vi "3.2.0_BOOST_MODE.vi"(6 "Data in":T2, 8 "error in (no error)":errorcluster, 9 "AllControls In":T1, 10 "?":T3, 11 "Message Queue out":T4) -> (0 "error out":errorcluster, 1 "Flow":string, 2 "Data":T3, 3 "Message Queue Out":T4, 4 "Data out":T2)   [LabVIEW 2017]
uses:
  Depends/AMC/subVIs/TypeDefs/amc_Message Queue.ctl
  Depends/AMC/subVIs/TypeDefs/amc_Message.ctl
  Depends/Tools/Keyed Array/Tools_KeyedArray KeyedArray.ctl
  Ctrls/Data.ctl
  Ctrls/CSV_Data.ctl
  Ctrls/AllControls.ctl
  DIPC 692 Daemon API/typdef/get_parameter.ctl
  Ctrls/AlarmIndex.ctl
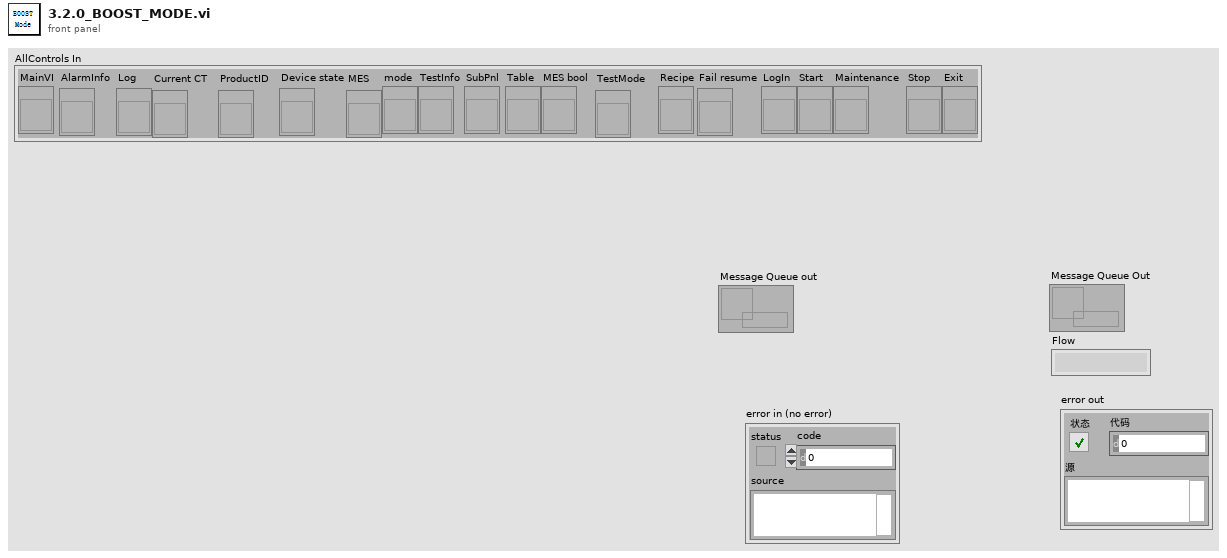
[diagram p1: front panel]
types:
  T1 = typedef "AllControls.ctl" = cluster{"MainVI":refnum<vi>, "AlarmInfo":refnum<vi>, "Log":refnum<vi>, "Current CT":refnum<vi>, "ProductID":refnum<vi>, "Device state":refnum<vi>, "MES":refnum<vi>, "mode":refnum<vi>, "TestInfo":refnum<vi>, "SubPnl":refnum<vi>, "Table":refnum<vi>, "MES bool":refnum<vi>, "TestMode":refnum<vi>, "Recipe":refnum<vi>, "Fail resume":refnum<vi>, "LogIn":refnum<vi>, "Start":refnum<vi>, "Maintenance":refnum<vi>, "Stop":refnum<vi>, "Exit":refnum<vi>}
  T2 = typedef "CSV_Data.ctl" = cluster{"Initialisation":cluster{"LMT - Connect UUT (con COM)":string, "LMT - Software Version (rrel)":string, "LMT - Write SKU file (wskuc)":string, "LMT - SKU file name":string, "Connect UUT DDM":string, "Read DDM EOL Timestamp - Mode":string, "Read DDM EOL Timestamp - Timestamp":string, "Read DDM EOL Timestamp - Rig ID":string, "Read DDM EOL Timestamp - Passmark ID":string, "Read DDM EOL Timestamp - Passmark Rev":string, "Software Version before flashing":string, "Read Hardware Serial":string, "UUT DDM SN":string, "Compare DDM SN with MES SN":string, "Backup PCBA Calibration EEPROM Response - CAL":string, "Flash Firmware Version":string, "Check SW Version":string, "Read DDM SW Version after flashing":string, "Set SKU Config":string, "Ready Status":string, "Set Device Mode to EOL":string, "DDM Parameter - Voltage":string, "DDM Parameter - Current":string, "DDM Parameter - Power":string, "DDM Parameter - Speed":string, "DDM Parameter - Pressure":string, "Tester Parameter - Voltage":string, "Tester Parameter - Current":string, "Tester Parameter - Power":string, "Tester Parameter - Ambient Pressure":string, "Tester Parameter - Ambient Temperature":string, "Calculated Parameter - DDM Pressure Corrected":string, "Calculated Parameter - DDM Real Power":string, "Calculated Parameter - Delta V":string}, "BEMF_Calibration":cluster{"Calibration Result - eol_cold_bemf_temp":string, "DDM Ambient Temp":string, "Restriction Plate Diameter":string, "Calibration Result - eol_bemf_mp_cold_coef_a":string, "Calibration Result - eol_bemf_mp_cold_coef_b":string, "Calibration Result - eol_bemf_mp_cold_coef_c":string, "Calibration Result - eol_bemf_lsi_cold_ref_coeffs":string, "Get - Calibration Result - eol_bemf_lsi_speed":string, "Get - Calibration Result - eol_bemf_lsi_integral_0":string, "Calibration Result - eol_bemf_lsi_integral_1":string, "Get - Calibration Result - eol_bemf_lsi_integral_2":string, "Get - Calibration Result - eol_cold_bemf":string, "Get - Calibration Result - eol_cold_bemf_fisf":string, "Finalise Calibration":string, "Compare -Calibration Result - eol_cold_bemf":string, "Compare -Calibration Result - eol_cold_bemf_fisf":string}, "ECO":cluster{"Reset Power Tune":string, "Reset BEMF FISF Calibration":string, "Restriction Plate Diameter":string, "ECO - Stabilisation Time":string, "ECO - DDM Parameter - Voltage":string, "ECO - DDM Parameter - Current":string, "ECO - DDM Parameter - Power":string, "ECO - DDM Parameter - Measured Power":string, "ECO - DDM Parameter - Speed":string, "ECO - DDM Parameter - Pressure":string, "ECO - Tester Parameter - Voltage":string, "ECO - Tester Parameter - Current":string, "ECO - Tester Parameter - Power":string, "ECO - Tester Parameter - Ambient Pressure":string, "ECO - Tester Parameter - Ambient Temperature":string, "ECO - Tester Parameter - Ambient Humidity":string, "ECO - Calculated Parameter - DDM Pressure Corrected":string, "ECO - Calculated Parameter - DDM Real Power":string, "ECO - Calculated Parameter - Delta V":string, "ECO - Calculated Parameter - Flowrate":string, "ECO - Calculated Parameter - Airwatt":string, "ECO - Formula":string, "PT ECO - Power Tune Mode Status":string}, "BOOST":cluster{"Restriction Plate Diameter":string, "BOOST - Stabilisation Time":string, "BOOST - DDM Parameter - Voltage":string, "BOOST - DDM Parameter - Current":string, "BOOST - DDM Parameter - Power":string, "BOOST - DDM Parameter - Measured Power":string, "BOOST - DDM Parameter - Speed":string, "BOOST - DDM Parameter - Pressure":string, "BOOST - Tester Parameter - Voltage":string, "BOOST - Tester Parameter - Current":string, "BOOST - Tester Parameter - Power":string, "BOOST - Tester Parameter - Ambient Pressure":string, "BOOST - Tester Parameter - Ambient Temperature":string, "BOOST - Tester Parameter - Ambient Humidity":string, "BOOST - Calculated Parameter - DDM Pressure Corrected":string, "BOOST - Calculated Parameter - DDM Real Power":string, "BOOST - Calculated Parameter - Delta V":string, "BOOST - Calculated Parameter - Flowrate":string, "BOOST - Calculated Parameter - Airwatt":string, "BOOST - Get AM Presence":string, "Air Muscle Turn Off Status":string, "BOOST - Air Muscle Calculated Parameter - Airwatt B":string, "BOOST - Air Muscle Calculate Airwatt Delta":string, "PT BOOST - Power Tune Mode Status":string, "Finalise Calibration":string, "ECO - Get AW Calibration value":string, "BOOST - Get AW Calibration value":string}, "MAX":cluster{"Restriction Plate Diameter":string, "MAX - Stabilisation Time":string, "Get Average Delta Tmag (LSIdelta_FISFdelta_LSItmag_FISFtmag_IIRtmag)":string, "Get Average Delta Tmag FISF":string, "MAX - DDM Parameter - Voltage":string, "MAX - DDM Parameter - Current":string, "MAX - DDM Parameter - Power":string, "MAX - DDM Parameter - Measured Power":string, "MAX - DDM Parameter - Speed":string, "MAX - DDM Parameter - Pressure":string, "MAX - Tester Parameter - Voltage":string, "MAX - Tester Parameter - Current":string, "MAX - Tester Parameter - Power":string, "MAX - Tester Parameter - Ambient Pressure":string, "MAX - Tester Parameter - Ambient Temperature":string, "MAX - Tester Parameter - Ambient Humidity":string, "MAX - Calculated Parameter - DDM Pressure Corrected":string, "MAX - Calculated Parameter - DDM Real Power":string, "MAX - Calculated Parameter - Delta V":string, "MAX - Calculated Parameter - Flowrate":string, "MAX - Calculated Parameter - Airwatt":string, "MAX_FISF_Check_Average_Delta_Tmag":string, "MAX - FISF - BEMF Finetune Result":string, "MAX tune - Delta P1":string, "MAX tune - Calculated Parameter - Airwatt":string, "Calculate Delta Airwatts - MAX finetune - Delta P2":string, "MAX finetune - DDM Parameter - Voltage":string, "MAX finetune - DDM Parameter - Current":string, "MAX finetune - DDM Parameter - Power":string, "MAX finetune - DDM Parameter - Measured Power":string, "MAX finetune - DDM Parameter - Speed":string, "MAX finetune - DDM Parameter - Pressure":string, "MAX finetune - Tester Parameter - Voltage":string, "MAX finetune - Tester Parameter - Current":string, "MAX finetune - Tester Parameter - Power":string, "MAX finetune - Tester Parameter - Ambient Pressure":string, "MAX finetune - Tester Parameter - Ambient Temperature":string, "MAX finetune - Tester Parameter - Ambient Humidity":string, "MAX finetune - Calculated Parameter - DDM Pressure Corrected":string, "MAX finetune - Calculated Parameter - DDM Real Power":string, "MAX finetune - Calculated Parameter - Delta V":string, "MAX finetune - Calculated Parameter - Flowrate":string, "MAX finetune - Calculated Parameter - Airwatt":string, "Check Derate Result":string, "Delta Tmag FISF":string, "Get Hot BEMF Result":string, "Calculate delta Pressure":string, "Finalise Calibration":string, "Calculate & Check Delta BEMF":string, "Delta P Airwatts Value":string}, "LL":cluster{"DDM Ambient Temp":string, "Restriction Plate Diameter":string, "LL - DDM Parameter - Voltage":string, "LL - DDM Parameter - Current":string, "LL - DDM Parameter - Power":string, "LL - DDM Parameter - Measured Power":string, "LL - DDM Parameter - Speed":string, "LL - DDM Parameter - Pressure":string, "LL - Tester Parameter - Voltage":string, "LL - Tester Parameter - Current":string, "LL - Tester Parameter - Power":string, "LL - DDM Real Power":string, "LL - Calibrate Task Detect LL":string}, "HL":cluster{"HL - DDM Parameter - Voltage":string, "HL - DDM Parameter - Current":string, "HL - DDM Parameter - Power":string, "HL - DDM Parameter - Measured Power":string, "HL - DDM Parameter - Speed":string, "HL - DDM Parameter - Pressure":string, "HL - Tester Parameter - Voltage":string, "HL - Tester Parameter - Current":string, "HL - Tester Parameter - Power":string, "HL - DDM Real Power":string, "HL - Calibrate Task Detect HL":string}, "LH":cluster{"Restriction Plate Diameter":string, "LH - DDM Parameter - Voltage":string, "LH - DDM Parameter - Current":string, "LH - DDM Parameter - Power":string, "LH - DDM Parameter - Measured Power":string, "LH - DDM Parameter - Speed":string, "LH - DDM Parameter - Pressure":string, "LH - Tester Parameter - Voltage":string, "LH - Tester Parameter - Current":string, "LH - Tester Parameter - Power":string, "LH - DDM Real Power":string, "LH - Calibrate Task Detect LH":string}, "HH":cluster{"HH - DDM Parameter - Voltage":string, "HH - DDM Parameter - Current":string, "HH - DDM Parameter - Power":string, "HH - DDM Parameter - Measured Power":string, "HH - DDM Parameter - Speed":string, "HH - DDM Parameter - Pressure":string, "HH - Tester Parameter - Voltage":string, "HH - Tester Parameter - Current":string, "HH - Tester Parameter - Power":string, "HH - DDM Real Power":string, "HH - Calibrate Task Detect HH":string}, "Inlet Blockage Calibration":cluster{"Inlet Blockage Calibration - DDM Parameter - Voltage":string, "Inlet Blockage Calibration - DDM Parameter - Current":string, "Inlet Blockage Calibration - DDM Parameter - Power":string, "Inlet Blockage Calibration - DDM Parameter - Measured Power":string, "Inlet Blockage Calibration - DDM Parameter - Speed":string, "Inlet Blockage Calibration - DDM Parameter - Pressure":string, "Inlet Blockage Calibration - Tester Parameter - Voltage":string, "Inlet Blockage Calibration - Tester Parameter - Current":string, "Inlet Blockage Calibration - Tester Parameter - Power":string, "Inlet Blockage Calibration - DDM Real Power":string, "Calibration Inlet Blockage_E":string, "Finalise Calibration":string, "Get Task Detect LL":string, "Get Task Detect HL":string, "Get Task Detect LH":string, "Get Task Detect HH":string, "Calibration Inlet Blockage":string, "Calibration eol cold bemf temp":string}, "GOOD":cluster{"GOOD UNIT - Clear EEPROM Error Log":string, "GOOD UNIT - Write Product Timestamp - Mode":string, "GOOD UNIT - Write Product Timestamp - Timestamp":string, "GOOD UNIT - Write Product Timestamp - Rig ID":string, "GOOD UNIT - Write Product Timestamp - Passmark ID":string, "GOOD UNIT - Write Product Timestamp - Passmark Rev":string, "GOOD UNIT - Set Device Mode to PROD":string, "GOOD UNIT - Backup PCBA Calibration EEPROM Response":string, "GOOD UNIT - Check Security Bit":string, "GOOD UNIT - Set Calibration Lock":string, "GOOD UNIT - Get_Calibration_Lock":string, "GOOD UNIT - Disconnect UUT":string}, "NG":cluster{"NG UNIT - Read NVM Error":string, "NG UNIT - Set Device Mode to FCT":string, "NG UNIT - Backup PCBA Calibration EEPROM Response - CAL":string, "NG UNIT - Backup PCBA Calibration EEPROM Response - ERROR":string, "NG UNIT - Backup PCBA Calibration EEPROM Response - USAGE":string, "NG UNIT - Disconnect UUT":string}, "SN":string, "Table":string[][], "Count":cluster{"Total":i32, "OK":i32, "NG":i32, "Yield":dbl}, "Start Time":timestamp, "daemon reference":refnum<k5>, "CT":dbl, "Config":string[][], "OK/NG":bool, "Station ID":string, "MES DDM SN":string, "MES PCBA SN":string, "Retest":string, "Variant":string, "Initialisation_Status":cluster{"LMT - Connect UUT (con COM)":string, "LMT - Software Version (rrel)":string, "LMT - Write SKU file (wskuc)":string, "LMT - SKU file name":string, "Connect UUT DDM":string, "Read DDM EOL Timestamp - Mode":string, "Read DDM EOL Timestamp - Timestamp":string, "Read DDM EOL Timestamp - Rig ID":string, "Read DDM EOL Timestamp - Passmark ID":string, "Read DDM EOL Timestamp - Passmark Rev":string, "Software Version before flashing":string, "Read Hardware Serial":string, "UUT DDM SN":string, "Compare DDM SN with MES SN":string, "Backup PCBA Calibration EEPROM Response - CAL":string, "Flash Firmware Version":string, "Check SW Version":string, "Read DDM SW Version after flashing":string, "Set SKU Config":string, "Ready Status":string, "Set Device Mode to EOL":string, "DDM Parameter - Voltage":string, "DDM Parameter - Current":string, "DDM Parameter - Power":string, "DDM Parameter - Speed":string, "DDM Parameter - Pressure":string, "Tester Parameter - Voltage":string, "Tester Parameter - Current":string, "Tester Parameter - Power":string, "Tester Parameter - Ambient Pressure":string, "Tester Parameter - Ambient Temperature":string, "Calculated Parameter - DDM Pressure Corrected":string, "Calculated Parameter - DDM Real Power":string, "Calculated Parameter - Delta V":string}, "BEMF_Calibration_Status":cluster{"Calibration Result - eol_cold_bemf_temp":string, "DDM Ambient Temp":string, "Restriction Plate Diameter":string, "Calibration Result - eol_bemf_mp_cold_coef_a":string, "Calibration Result - eol_bemf_mp_cold_coef_b":string, "Calibration Result - eol_bemf_mp_cold_coef_c":string, "Calibration Result - eol_bemf_lsi_cold_ref_coeffs":string, "Get - Calibration Result - eol_bemf_lsi_speed":string, "Get - Calibration Result - eol_bemf_lsi_integral_0":string, "Calibration Result - eol_bemf_lsi_integral_1":string, "Get - Calibration Result - eol_bemf_lsi_integral_2":string, "Get - Calibration Result - eol_cold_bemf":string, "Get - Calibration Result - eol_cold_bemf_fisf":string, "Finalise Calibration":string, "Compare -Calibration Result - eol_cold_bemf":string, "Compare -Calibration Result - eol_cold_bemf_fisf":string}, "ECO_Status":cluster{"Reset Power Tune":string, "Reset BEMF FISF Calibration":string, "Restriction Plate Diameter":string, "ECO - Stabilisation Time":string, "ECO - DDM Parameter - Voltage":string, "ECO - DDM Parameter - Current":string, "ECO - DDM Parameter - Power":string, "ECO - DDM Parameter - Measured Power":string, "ECO - DDM Parameter - Speed":string, "ECO - DDM Parameter - Pressure":string, "ECO - Tester Parameter - Voltage":string, "ECO - Tester Parameter - Current":string, "ECO - Tester Parameter - Power":string, "ECO - Tester Parameter - Ambient Pressure":string, "ECO - Tester Parameter - Ambient Temperature":string, "ECO - Tester Parameter - Ambient Humidity":string, "ECO - Calculated Parameter - DDM Pressure Corrected":string, "ECO - Calculated Parameter - DDM Real Power":string, "ECO - Calculated Parameter - Delta V":string, "ECO - Calculated Parameter - Flowrate":string, "ECO - Calculated Parameter - Airwatt":string, "ECO - Formula":string, "PT ECO - Power Tune Mode Status":string}, "BOOST_Status":cluster{"Restriction Plate Diameter":string, "BOOST - Stabilisation Time":string, "BOOST - DDM Parameter - Voltage":string, "BOOST - DDM Parameter - Current":string, "BOOST - DDM Parameter - Power":string, "BOOST - DDM Parameter - Measured Power":string, "BOOST - DDM Parameter - Speed":string, "BOOST - DDM Parameter - Pressure":string, "BOOST - Tester Parameter - Voltage":string, "BOOST - Tester Parameter - Current":string, "BOOST - Tester Parameter - Power":string, "BOOST - Tester Parameter - Ambient Pressure":string, "BOOST - Tester Parameter - Ambient Temperature":string, "BOOST - Tester Parameter - Ambient Humidity":string, "BOOST - Calculated Parameter - DDM Pressure Corrected":string, "BOOST - Calculated Parameter - DDM Real Power":string, "BOOST - Calculated Parameter - Delta V":string, "BOOST - Calculated Parameter - Flowrate":string, "BOOST - Calculated Parameter - Airwatt":string, "BOOST - Get AM Presence":string, "Air Muscle Turn Off Status":string, "BOOST - Air Muscle Calculated Parameter - Airwatt B":string, "BOOST - Air Muscle Calculate Airwatt Delta":string, "PT BOOST - Power Tune Mode Status":string, "Finalise Calibration":string, "ECO - Get AW Calibration value":string, "BOOST - Get AW Calibration value":string}, "MAX_Status":cluster{"Restriction Plate Diameter":string, "MAX - Stabilisation Time":string, "Get Average Delta Tmag (LSIdelta_FISFdelta_LSItmag_FISFtmag_IIRtmag)":string, "Get Average Delta Tmag FISF":string, "MAX - DDM Parameter - Voltage":string, "MAX - DDM Parameter - Current":string, "MAX - DDM Parameter - Power":string, "MAX - DDM Parameter - Measured Power":string, "MAX - DDM Parameter - Speed":string, "MAX - DDM Parameter - Pressure":string, "MAX - Tester Parameter - Voltage":string, "MAX - Tester Parameter - Current":string, "MAX - Tester Parameter - Power":string, "MAX - Tester Parameter - Ambient Pressure":string, "MAX - Tester Parameter - Ambient Temperature":string, "MAX - Tester Parameter - Ambient Humidity":string, "MAX - Calculated Parameter - DDM Pressure Corrected":string, "MAX - Calculated Parameter - DDM Real Power":string, "MAX - Calculated Parameter - Delta V":string, "MAX - Calculated Parameter - Flowrate":string, "MAX - Calculated Parameter - Airwatt":string, "MAX_FISF_Check_Average_Delta_Tmag":string, "MAX - FISF - BEMF Finetune Result":string, "MAX tune - Delta P1":string, "MAX tune - Calculated Parameter - Airwatt":string, "Calculate Delta Airwatts - MAX finetune - Delta P2":string, "MAX finetune - DDM Parameter - Voltage":string, "MAX finetune - DDM Parameter - Current":string, "MAX finetune - DDM Parameter - Power":string, "MAX finetune - DDM Parameter - Measured Power":string, "MAX finetune - DDM Parameter - Speed":string, "MAX finetune - DDM Parameter - Pressure":string, "MAX finetune - Tester Parameter - Voltage":string, "MAX finetune - Tester Parameter - Current":string, "MAX finetune - Tester Parameter - Power":string, "MAX finetune - Tester Parameter - Ambient Pressure":string, "MAX finetune - Tester Parameter - Ambient Temperature":string, "MAX finetune - Tester Parameter - Ambient Humidity":string, "MAX finetune - Calculated Parameter - DDM Pressure Corrected":string, "MAX finetune - Calculated Parameter - DDM Real Power":string, "MAX finetune - Calculated Parameter - Delta V":string, "MAX finetune - Calculated Parameter - Flowrate":string, "MAX finetune - Calculated Parameter - Airwatt":string, "Check Derate Result":string, "Delta Tmag FISF":string, "Get Hot BEMF Result":string, "Calculate delta Pressure":string, "Finalise Calibration":string, "Calculate & Check Delta BEMF":string, "Delta P Airwatts Value":string}, "LL_Status":cluster{"DDM Ambient Temp":string, "Restriction Plate Diameter":string, "LL - DDM Parameter - Voltage":string, "LL - DDM Parameter - Current":string, "LL - DDM Parameter - Power":string, "LL - DDM Parameter - Measured Power":string, "LL - DDM Parameter - Speed":string, "LL - DDM Parameter - Pressure":string, "LL - Tester Parameter - Voltage":string, "LL - Tester Parameter - Current":string, "LL - Tester Parameter - Power":string, "LL - DDM Real Power":string, "LL - Calibrate Task Detect LL":string}, "HL_Status":cluster{"HL - DDM Parameter - Voltage":string, "HL - DDM Parameter - Current":string, "HL - DDM Parameter - Power":string, "HL - DDM Parameter - Measured Power":string, "HL - DDM Parameter - Speed":string, "HL - DDM Parameter - Pressure":string, "HL - Tester Parameter - Voltage":string, "HL - Tester Parameter - Current":string, "HL - Tester Parameter - Power":string, "HL - DDM Real Power":string, "HL - Calibrate Task Detect HL":string}, "LH_Status":cluster{"Restriction Plate Diameter":string, "LH - DDM Parameter - Voltage":string, "LH - DDM Parameter - Current":string, "LH - DDM Parameter - Power":string, "LH - DDM Parameter - Measured Power":string, "LH - DDM Parameter - Speed":string, "LH - DDM Parameter - Pressure":string, "LH - Tester Parameter - Voltage":string, "LH - Tester Parameter - Current":string, "LH - Tester Parameter - Power":string, "LH - DDM Real Power":string, "LH - Calibrate Task Detect LH":string}, "HH_Status":cluster{"HH - DDM Parameter - Voltage":string, "HH - DDM Parameter - Current":string, "HH - DDM Parameter - Power":string, "HH - DDM Parameter - Measured Power":string, "HH - DDM Parameter - Speed":string, "HH - DDM Parameter - Pressure":string, "HH - Tester Parameter - Voltage":string, "HH - Tester Parameter - Current":string, "HH - Tester Parameter - Power":string, "HH - DDM Real Power":string, "HH - Calibrate Task Detect HH":string}, "Inlet Blockage Calibration_Status":cluster{"Inlet Blockage Calibration - DDM Parameter - Voltage":string, "Inlet Blockage Calibration - DDM Parameter - Current":string, "Inlet Blockage Calibration - DDM Parameter - Power":string, "Inlet Blockage Calibration - DDM Parameter - Measured Power":string, "Inlet Blockage Calibration - DDM Parameter - Speed":string, "Inlet Blockage Calibration - DDM Parameter - Pressure":string, "Inlet Blockage Calibration - Tester Parameter - Voltage":string, "Inlet Blockage Calibration - Tester Parameter - Current":string, "Inlet Blockage Calibration - Tester Parameter - Power":string, "Inlet Blockage Calibration - DDM Real Power":string, "Calibration Inlet Blockage_E":string, "Finalise Calibration":string, "Get Task Detect LL":string, "Get Task Detect HL":string, "Get Task Detect LH":string, "Get Task Detect HH":string, "Calibration Inlet Blockage":string, "Calibration eol cold bemf temp":string}, "GOOD_Status":cluster{"GOOD UNIT - Clear EEPROM Error Log":string, "GOOD UNIT - Write Product Timestamp - Mode":string, "GOOD UNIT - Write Product Timestamp - Timestamp":string, "GOOD UNIT - Write Product Timestamp - Rig ID":string, "GOOD UNIT - Write Product Timestamp - Passmark ID":string, "GOOD UNIT - Write Product Timestamp - Passmark Rev":string, "GOOD UNIT - Set Device Mode to PROD":string, "GOOD UNIT - Backup PCBA Calibration EEPROM Response":string, "GOOD UNIT - Check Security Bit":string, "GOOD UNIT - Set Calibration Lock":string, "GOOD UNIT - Get_Calibration_Lock":string, "GOOD UNIT - Disconnect UUT":string}, "NG_Status":cluster{"NG UNIT - Read NVM Error":string, "NG UNIT - Set Device Mode to FCT":string, "NG UNIT - Backup PCBA Calibration EEPROM Response - CAL":string, "NG UNIT - Backup PCBA Calibration EEPROM Response - ERROR":string, "NG UNIT - Backup PCBA Calibration EEPROM Response - USAGE":string, "NG UNIT - Disconnect UUT":string}, "SKU":string, "Plate_Diameter":string, "Alarm":string}
  T3 = typedef "Data.ctl" = cluster{"Initialisation":cluster{"DDM_Parameter":dbl[], "DDM_Parameter_status":bool[], "Get_Tester_Parameter":dbl[], "Get_Tester_Parameter_status":bool[], "Cal_Tester_Parameter":dbl[], "Cal_Tester_Parameter_status":bool[], "sw_version_before_status":bool, "sw_version_after_status":bool, "Set_SKU_Config_With_LMT_status":bool, "FCT_timestamp_status":bool, "LMT_Connect_to_UUT_status":bool}, "BEMF_Calibration":cluster{"Read_ambient_temperature":dbl, "Calibration_Vaule":dbl[], "Calibration_Vaule _B":dbl[], "Calibration_Vaule_status":bool[], "Calibration_Vaule_B_status":bool[]}, "ECO":cluster{"DDM_Parameter":dbl[], "DDM_Parameter_status":bool[], "Get_Tester_Parameter":dbl[], "Get_Tester_Parameter_status":bool[], "Cal_Tester_Parameter":dbl[], "Cal_Tester_Parameter_status":bool[], "DDM_Parameter_after_power_tune":dbl[], "Get_Tester_Parameter_after_power_tune":dbl[], "Cal_Tester_Parameter_after_power_tune":dbl[], "Cal_Tester_Parameter_after_power_tune_status":bool[], "Delta_P":dbl}, "BOOST":cluster{"DDM_Parameter":dbl[], "DDM_Parameter_status":bool[], "Get_Tester_Parameter":dbl[], "Get_Tester_Parameter_status":bool[], "Cal_Tester_Parameter":dbl[], "Cal_Tester_Parameter_status":bool[], "DDM_Parameter_after_power_tune":dbl[], "Get_Tester_Parameter_after_power_tune":dbl[], "Cal_Tester_Parameter_after_power_tune":dbl[], "Cal_Tester_Parameter_after_power_tune_status":bool[], "airwatts_am_off":dbl, "AW_Delta_(AM_on_and_off)":dbl, "AW_Delta_(AM_on_and_off)_Status":bool, "Delta_P":dbl}, "MAX":cluster{"Average_Tmag_Data":cluster{"LSI Delta in degC":dbl, "FISF Delta in degc":dbl, "LSI Tmag in degC":dbl, "Fisf Tmag in degC":dbl, "IIR Tmag in degC":dbl}, "DDM_Parameter":dbl[], "DDM_Parameter_status":bool[], "Get_Tester_Parameter":dbl[], "Get_Tester_Parameter_status":bool[], "Cal_Tester_Parameter":dbl[], "BEMF_Finetune":cluster{"eol_bemf_mp_cold_coef_c":dbl, "eol_cold_bemf_fisf_offset":dbl}, "AW_Tune":cluster{"delta_P1":dbl, "delta_P_Setting":dbl}, "DDM_Parameter_after_Airwatts_Tune":dbl[], "Get_Tester_Parameter_after_Airwatts_Tune":dbl[], "Cal_Tester_Parameter_after_Airwatts_Tune":dbl[], "DDM_Parameter_after_Airwatts_Finetune":dbl[], "Get_Tester_Parameter_after_Airwatts_Finetune":dbl[], "Cal_Tester_Parameter_after_Airwatts_Finetune":dbl[], "AW_Finetune":cluster{"delta_P2":dbl, "delta_P_Setting":dbl}, "Delta_Tmag_after_tune":cluster{"LSI Delta in degC":dbl, "FISF Delta in degc":dbl, "LSI Tmag in degC":dbl, "Fisf Tmag in degC":dbl, "IIR Tmag in degC":dbl}, "Hot Bemf in mV":dbl, "DDM_Pressure":dbl, "Delta_Pressure":dbl, " Cold Bemf in mV":dbl, " delta Bemf":dbl, " delta p":dbl, "Delta_Pressure_status":bool, " delta Bemf_status":bool, "LSI Delta in degC_status":bool, "FISF Delta in degc_status":bool, "Max_check_derate_status_status":bool, "Average_All_data":dbl[][], "Average_Tmag_Data_status":bool[], "Average_Tmag_Data_after_tune_status":bool[], "Cal_Tester_Parameter_status":bool[], "Cal_Tester_Parameter_status_after_Airwatts_Tune":bool[], "Cal_Tester_Parameter_status_after_Airwatts_FineTune":bool[]}, "Task_Detect_Calib":cluster{"LL":cluster{"DDM_Parameter":dbl[], "DDM_Parameter_status":bool[], "Get_Tester_Parameter":dbl[], "Get_Tester_Parameter_status":bool[], "Set_task_detect_A":dbl, "Set_task_detect_A_Status":bool}, "HL":cluster{"DDM_Parameter":dbl[], "DDM_Parameter_status":bool[], "Get_Tester_Parameter":dbl[], "Get_Tester_Parameter_status":bool[], "Set_task_detect_B":dbl, "Set_task_detect_B_Status":bool}, "LH":cluster{"DDM_Parameter":dbl[], "DDM_Parameter_status":bool[], "Get_Tester_Parameter":dbl[], "Get_Tester_Parameter_status":bool[], "Set_task_detect_C":dbl, "Set_task_detect_C_Status":bool}, "HH":cluster{"DDM_Parameter":dbl[], "DDM_Parameter_status":bool[], "Get_Tester_Parameter":dbl[], "Get_Tester_Parameter_status":bool[], "Set_task_detect_D":dbl, "Read_and_check_calibration_Status":bool[], "Set_task_detect_D_Status":bool}, "Get_eol_inlet_blockage_E":dbl, "Calib_vaule":cluster{"Get_task_detect_LL":dbl, "Get_task_detect_HL":dbl, "Get_task_detect_LH":dbl, "Get_task_detect_HH":dbl, "eol_inlet_blockage":dbl, "eol_code_bemf_temp":dbl}, "calibrated temp":dbl, "Inlet_Blockage_Calibration":cluster{"DDM_Parameter":dbl[], "DDM_Parameter_status":bool[], "Get_Tester_Parameter":dbl[], "Get_Tester_Parameter_status":bool[]}, "Get_eol_inlet_blockage_E_Status":bool}, "good":cluster{"Write_Product_TS":cluster{"TIMESTAMP":i64, "RIG_ID":i64, "PASSMARK_ID":i64, "PASSMARK_REV":i64}, "Read_Product_TS":cluster{"TIMESTAMP":i64, "RIG_ID":i64, "PASSMARK_ID":i64, "PASSMARK_REV":i64}, "Good_Check_Secuity_Bit_Stauts":bool}}
  T4 = typedef "amc_Message Queue.ctl" = refnum<queue>
  T5 = typedef "HD Config.ctl" = cluster{" PC":cluster{"PC Address":u8[], "PC Port":i32}, "FCO":cluster{"COM":refnum<visa-resource-name>, "Baudrate":u32}, "DC Power ":cluster{"COM":refnum<visa-resource-name>, "Baudrate":u32}, "PW3336":cluster{"COM":refnum<visa-resource-name>, "Baudrate":u32}, "Lefoo":cluster{"COM":refnum<visa-resource-name>, "Baudrate":u32}, "AI Model":cluster{"COM":refnum<visa-resource-name>, "Baudrate":u32}, "DIPC":cluster{"COM":refnum<visa-resource-name>}, "NFC":cluster{"IP Address":string, "Port":u16, "Retry":u16}, "Motor":cluster{"COM":refnum<visa-resource-name>, "Baudrate":u32}, "Fail_resume_mode":bool, "GRR":bool}
  T6 = typedef "AlarmIndex.ctl" = enum16{"E-Stop", "Safety light grid", "UUT Sealing Cylinder HomePoint", "UUT Sealing Cylinder WorkPoint", "Orifice fixed Cylinder L HomePoint", "Orifice fixed Cylinder L WorkPoint", "Orifice fixed Cylinder R HomePoint", "Orifice fixed Cylinder R WorkPoint", "UUT Cylinder HomePoint", "UUT Cylinder WorkPoint", "Carrier fixed Cylinder L HomePoint", "Carrier fixed Cylinder L WorkPoint", "Carrier fixed Cylinder R HomePoint", "Carrier fixed Cylinder R WorkPoint", "Probe Cylinder HomePoint", "Probe Cylinder WorkPoint", "Motor Error", "Test Error"}
  T7 = typedef "get_parameter.ctl" = string
  T8 = typedef "Position Config.ctl" = cluster{"OrificeSize_12.7":i32, "OrificeSize_13":i32, "OrificeSize_30":i32, "OrificeSize_16":i32}
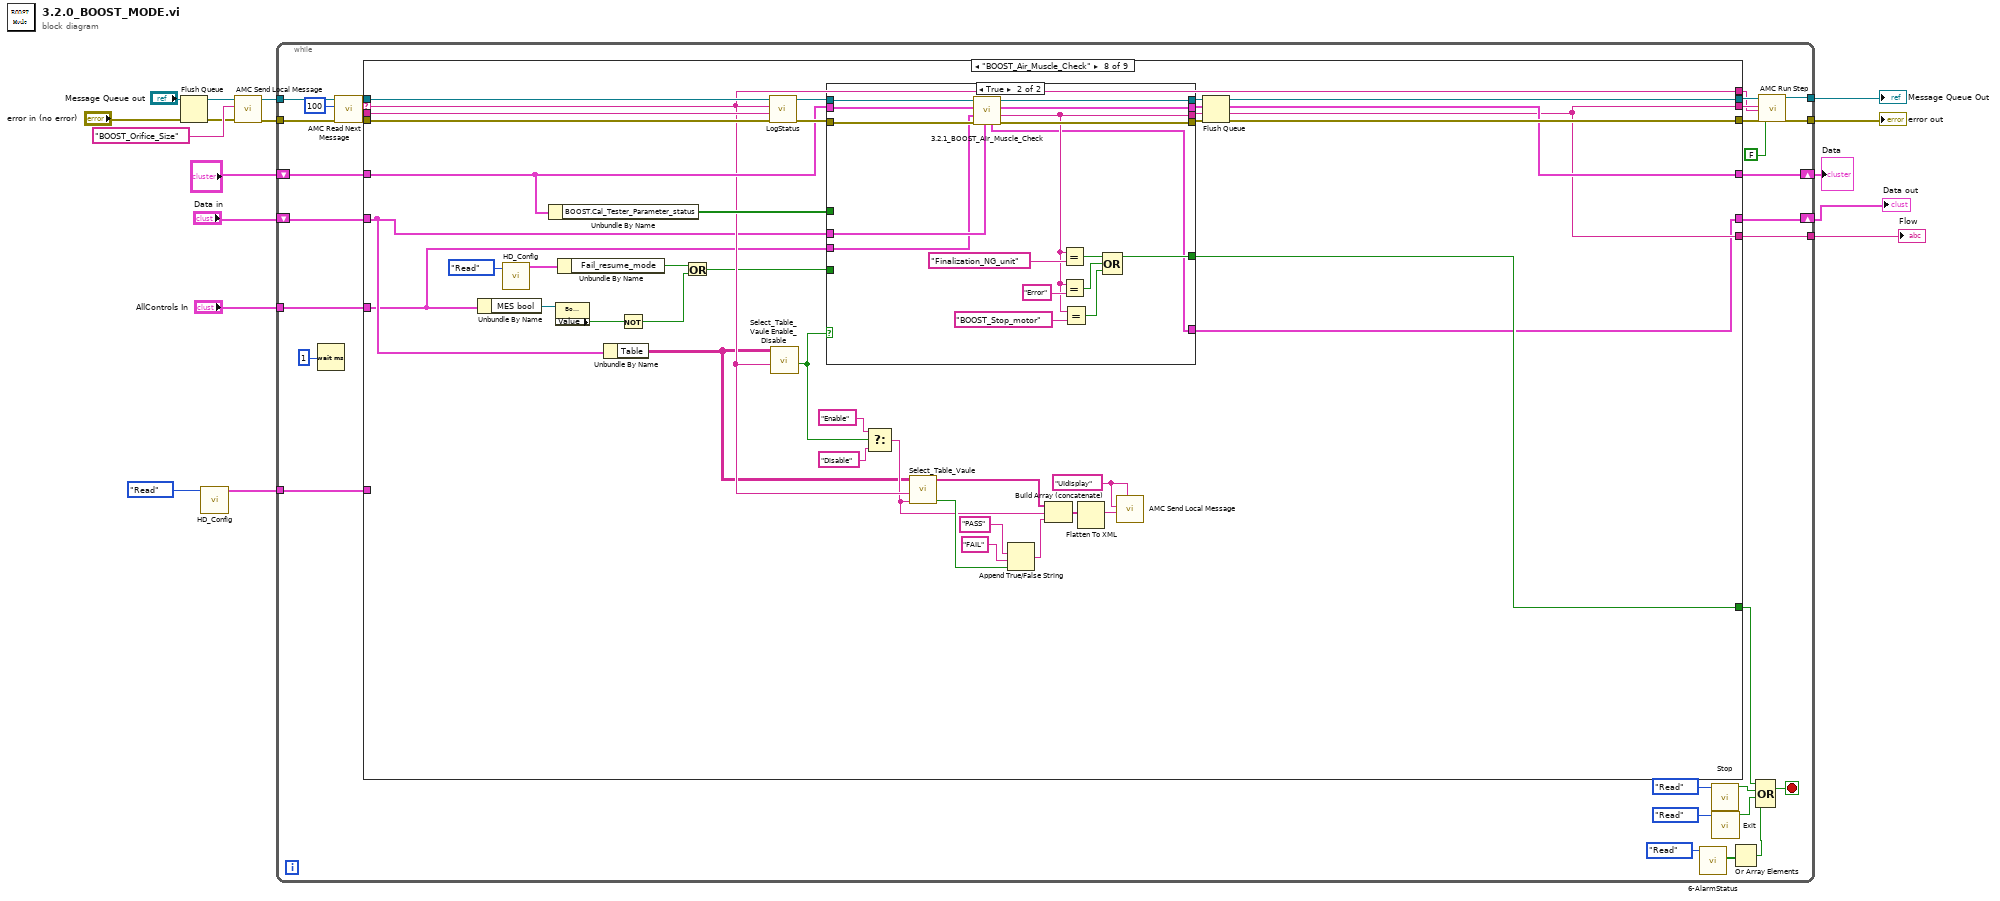
[diagram p0: block diagram]
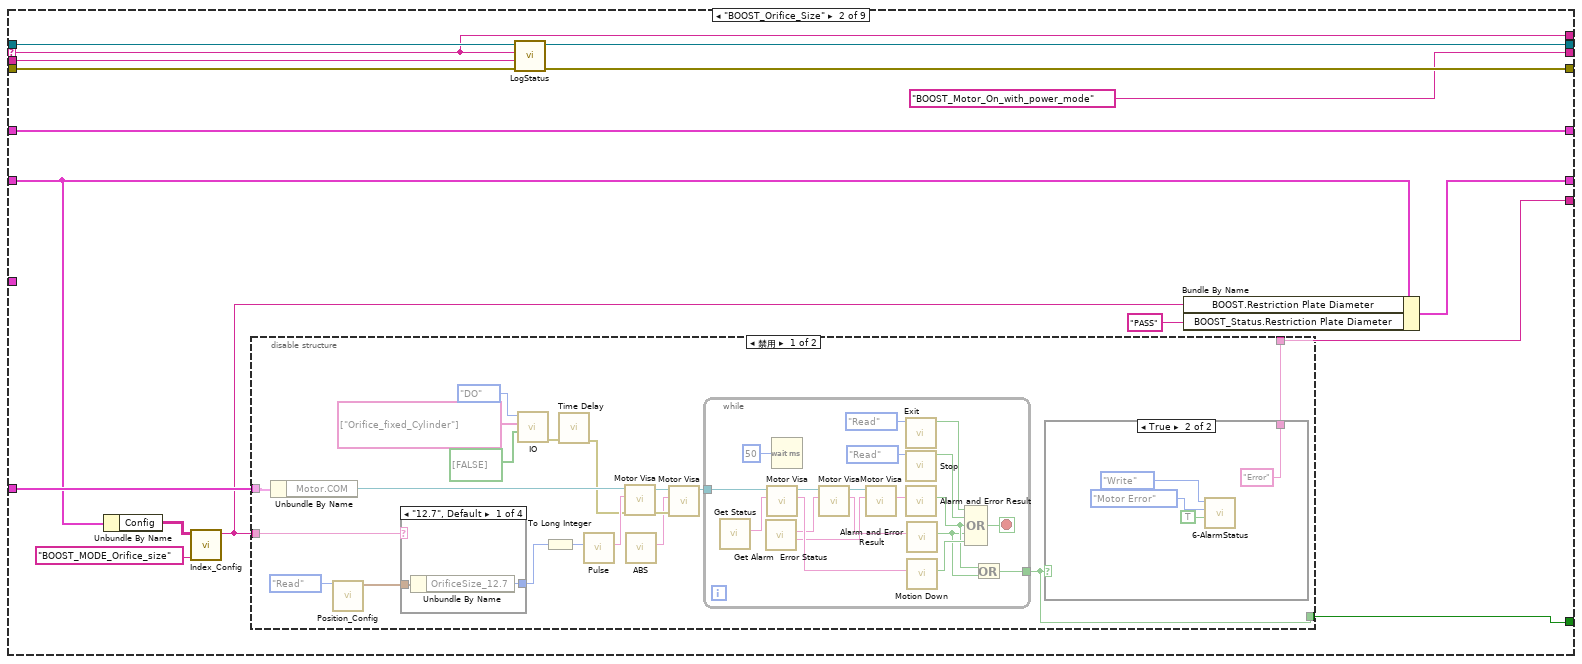
[diagram p3: hidden frame]
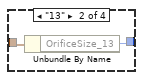
[diagram p4: hidden frame]
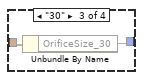
[diagram p5: hidden frame]
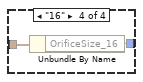
[diagram p6: hidden frame]
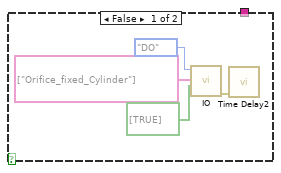
[diagram p7: hidden frame]
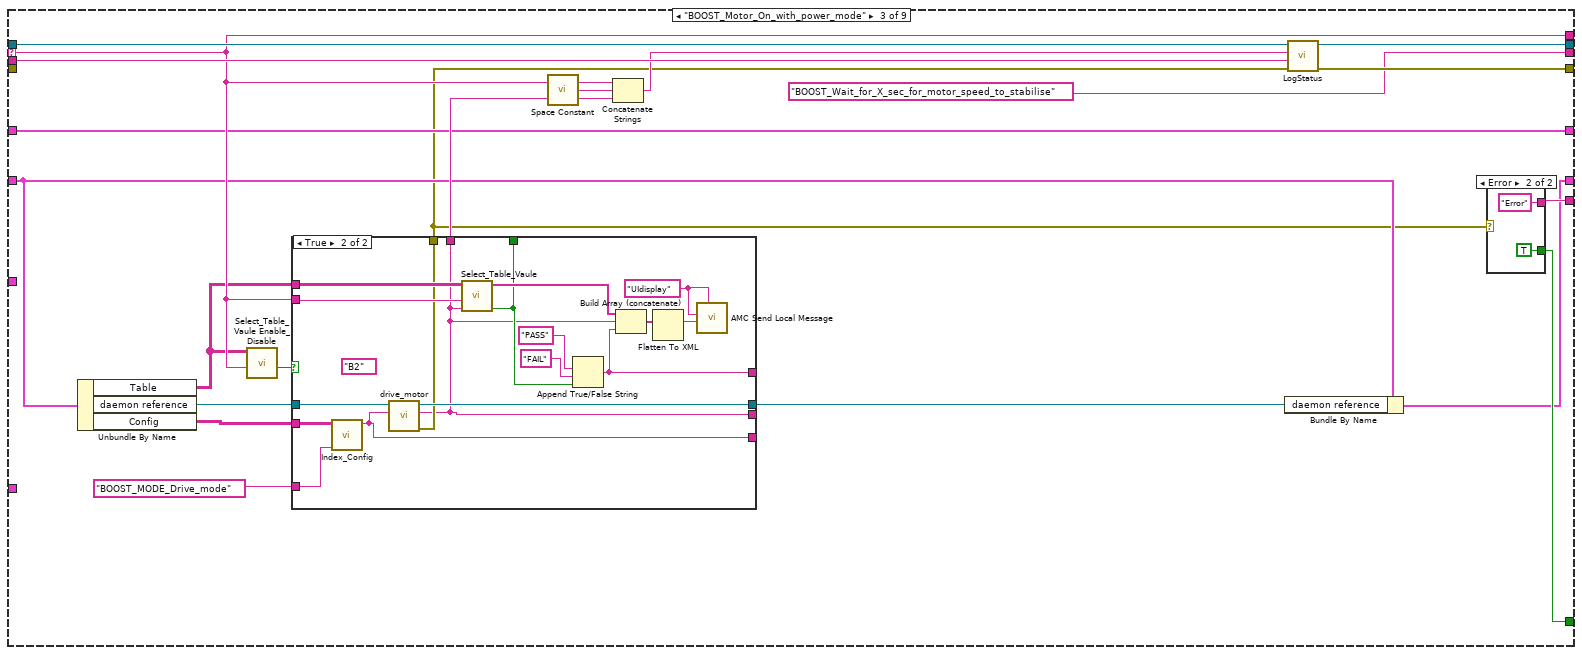
[diagram p9: hidden frame]
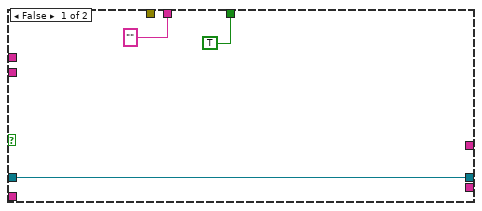
[diagram p11: hidden frame]
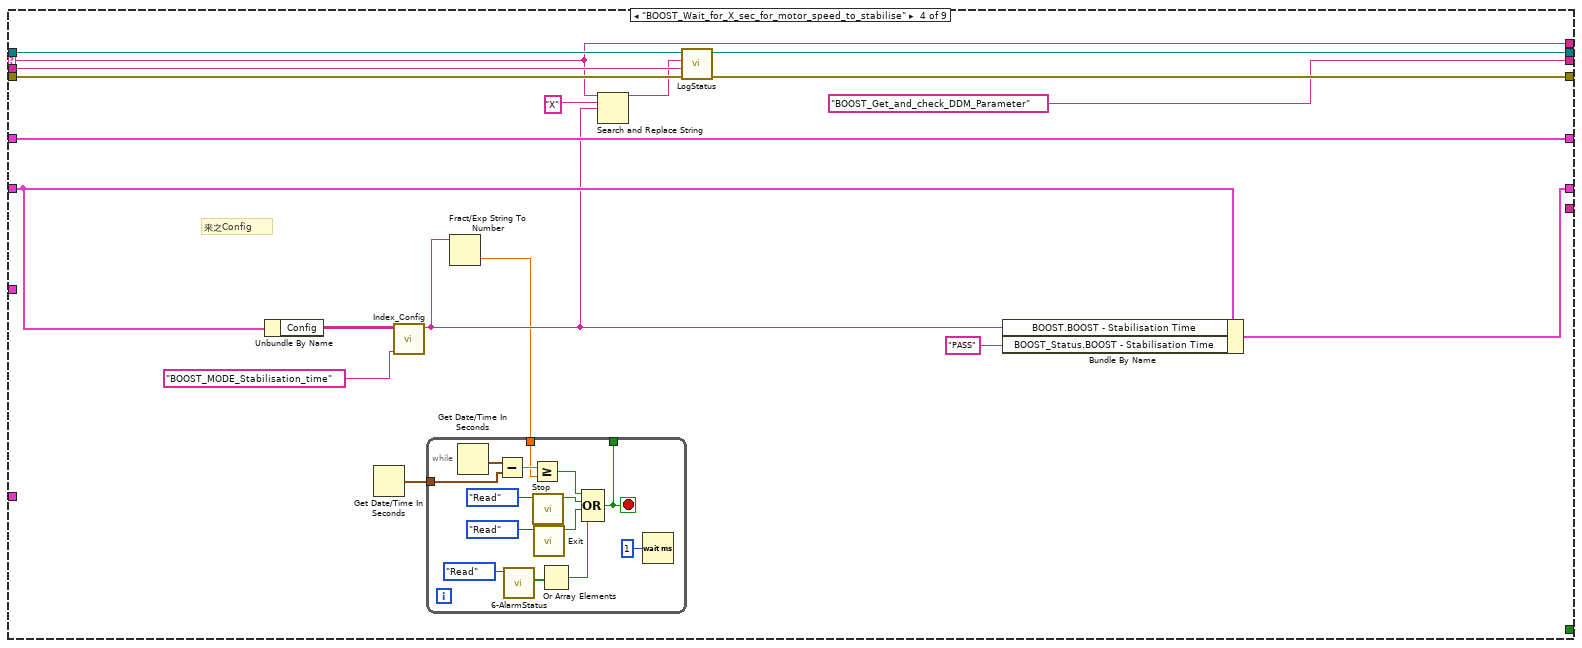
[diagram p12: hidden frame]
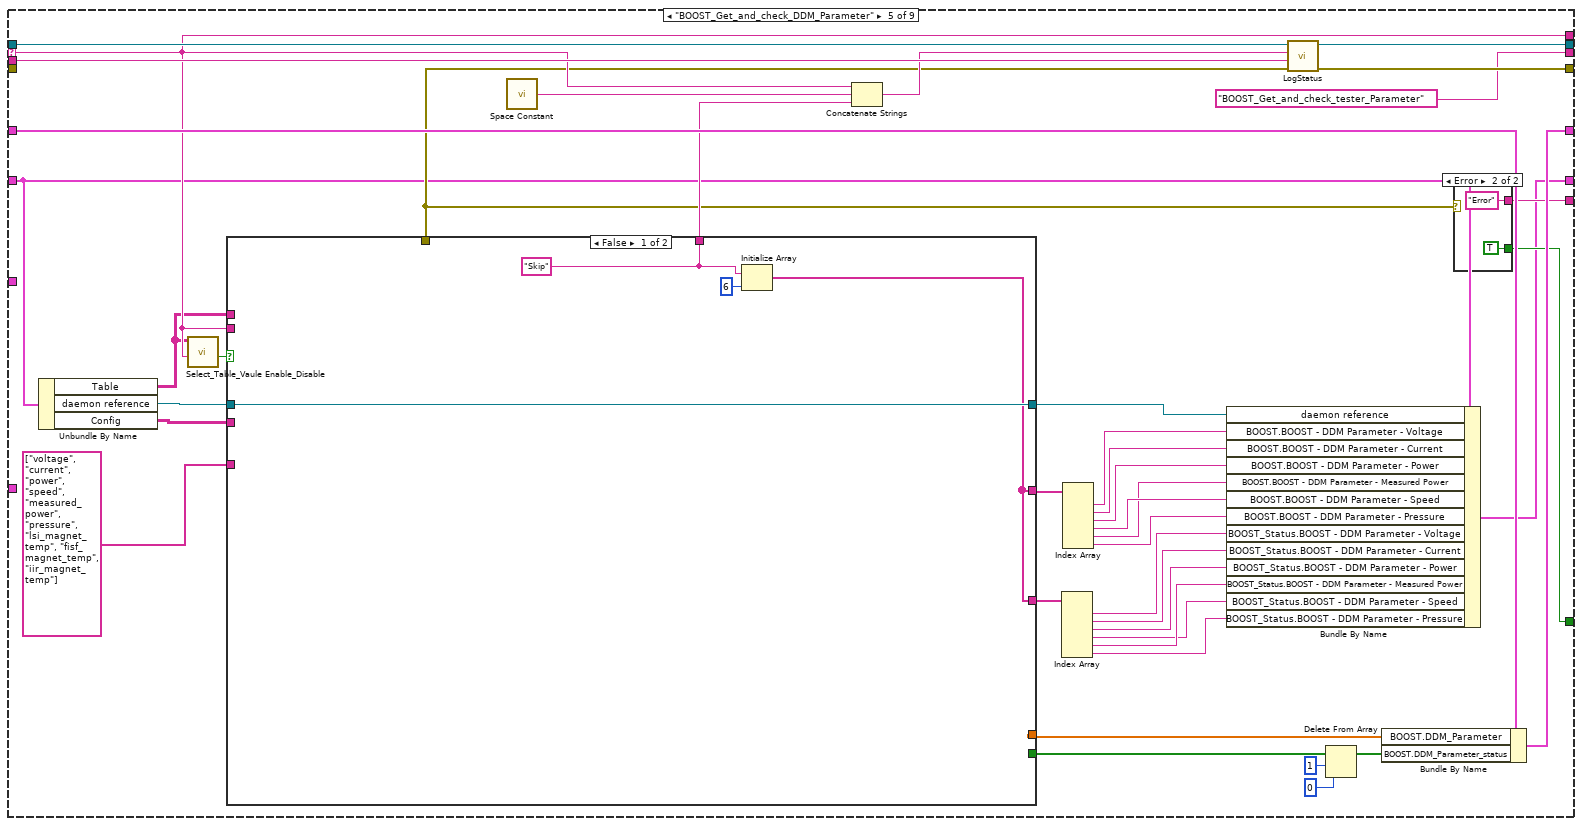
[diagram p13: hidden frame]
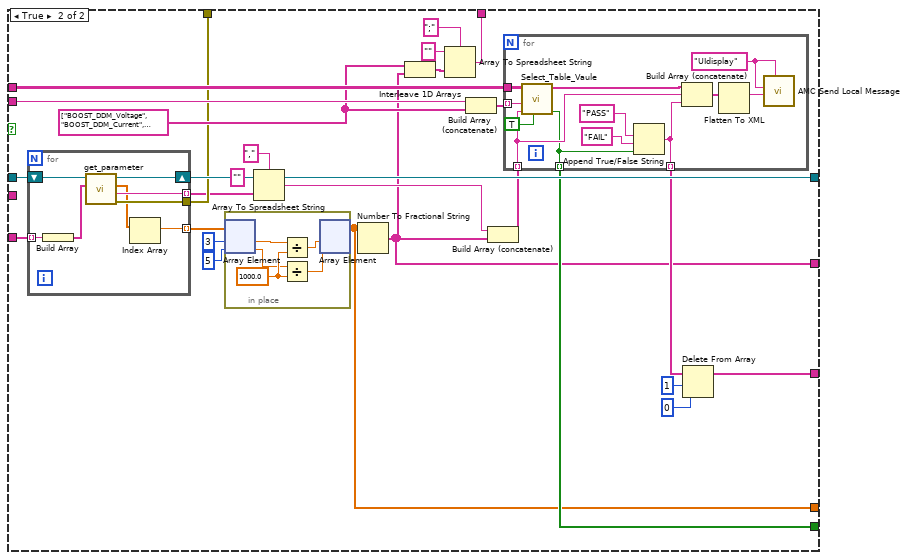
[diagram p15: hidden frame]
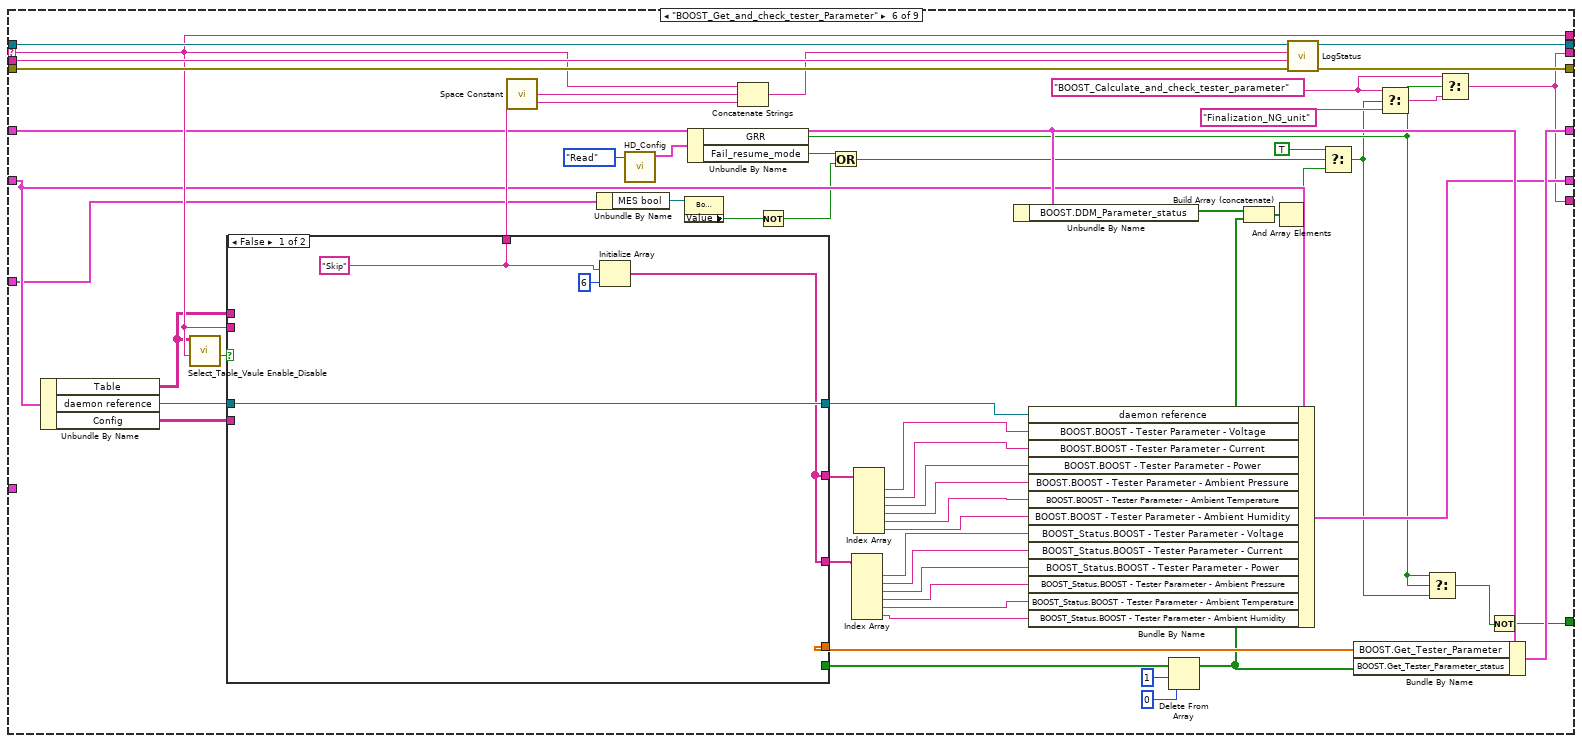
[diagram p16: hidden frame]
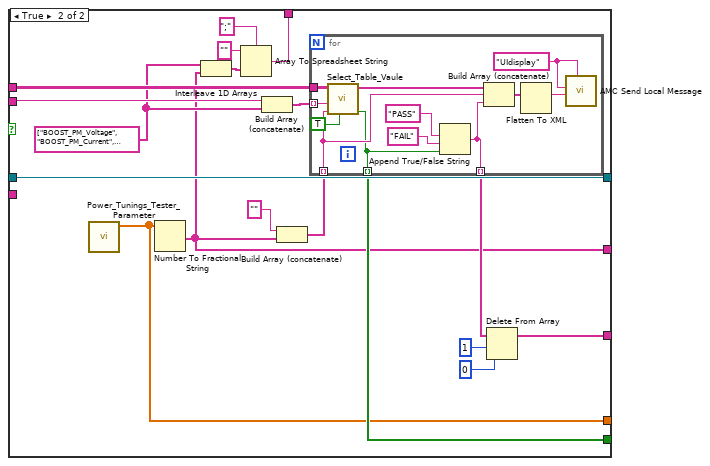
[diagram p17: hidden frame]
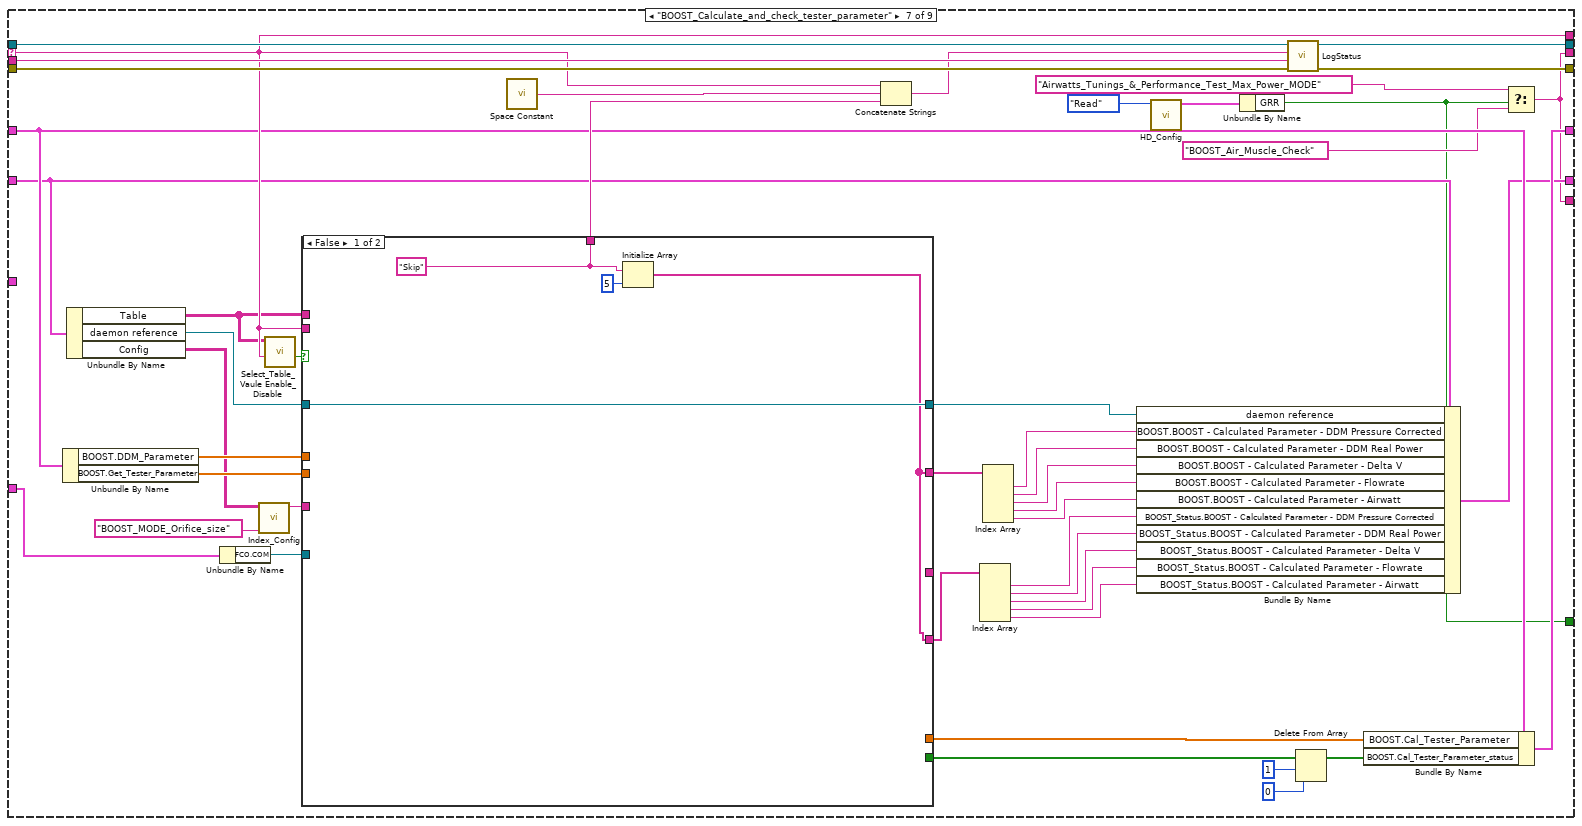
[diagram p18: hidden frame]
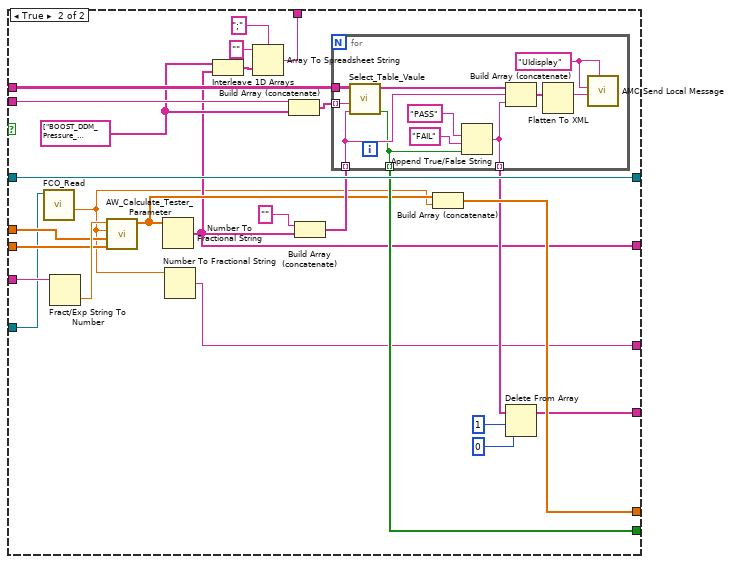
[diagram p19: hidden frame]
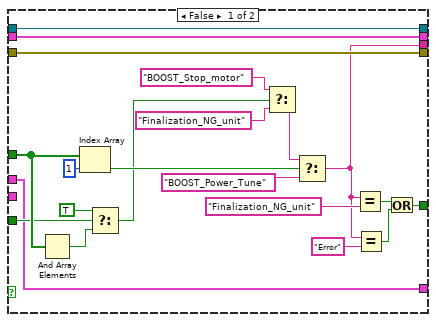
[diagram p20: hidden frame]
diagram:
  n1 = Flush Queue(queue="Message Queue out") -> (queue out=w4:T4)  [unwired: 1 in, 2 out]
  n2 = call "HD_Config.vi"("Step"=enum16{"Initial", "Write", "Read"}."Read") -> ("HD Config out"=w8:T5)  [unwired: 9 in, 1 out]
  n3 = call "AMC Send Local Message.vi"("error in (no error)"="error in (no error)", "Message Name"="BOOST_Orifice_Size", "Message Queue in"=w4) -> ("error out"=w13:errorcluster, "Message Queue out"=w14:T4)  [unwired: 7 in]
  n4 = while {
    tunnel: w14 -> [w47]
    tunnel: [w43] -> w6
    tunnel: w13 -> [w41]
    tunnel: [w38] -> w5
    shift-right: [w34] -> w10
    shift-left: "?" -> [w35]
    tunnel: w8 -> [w33]
    tunnel: [w29] -> w7
    shift-right: [w20] -> w1
    shift-left: "Data in" -> [w22]
    tunnel: "AllControls In" -> [w21]
    stop <- w23 stop-if-true
    n5 = Wait (ms)(milliseconds to wait=u32 1 ("等待时间（毫秒）")) -> ()  [unwired: 1 out]
    n6 = call "AMC Read Next Message.vi"("error in (no error)"=w41, "timeout (1ms)"=100, "Message Queue in"=w47) -> ("error out"=w40:errorcluster, "Message Value"=w31:string, "Message Name"=w45:string, "Message Queue out"=w46:T4)  [unwired: 1 in, 4 out]
    n7 = case shown="\"BOOST_Air_Muscle_Check\"" w45 {
      selector: w45 -> [_ w63 w134 w174 w225 w339 w420 w486 w560]
      tunnel: w46 -> [w51 w67 w141 w180 w234 w348 w428 w501 w574]
      tunnel: [w51 w67 w141 w180 w234 w348 w428 w481 w554] -> w44
      tunnel: w40 -> [w50 w66 _ w179 _ w347 w427 w505 w578]
      tunnel: [w50 w65 w140 w178 w233 w346 w426 w502 w575] -> w39
      tunnel: [_ w60 w128 _ w214 w331 w394 w496 TRUE] -> w24
      tunnel: w35 -> [w49 w56 w126 w170 w230 w334 w417 w497 w570]
      tunnel: [w49 w56 w126 w170 w229 w343 w424 w499 w572] -> w34
      tunnel: w31 -> [_ w64 w139 w177 w232 w345 w425 w504 w577]
      tunnel: [_ w63 w134 w174 w225 w339 w420 w486 w560] -> w30
      tunnel: w33 -> [_ w61 _ _ _ _ w407 _ _]
      tunnel: [_ "BOOST_Motor_On_with_power_mode" "BOOST_Wait_for_X_sec_for_motor_speed_to_stabilise" "BOOST_Get_and_check_DDM_Parameter" "BOOST_Get_and_check_tester_Parameter" w310 w395 w498 w571] -> w32
      tunnel: [_ w59 w129 _ w215 w310 w395 w498 w571] -> w29
      tunnel: w22 -> [w48 w53 w125 w169 w211 w325 w403 w472 w546]
      tunnel: w21 -> [_ _ _ _ _ w313 _ w470 w544]
      tunnel: [w48 w55 w123 w168 w209 w322 w402 w471 w545] -> w20
      frame "假", Default {
      }
      frame "BOOST_Orifice_Size" {
        n8 = Unbundle By Name(w53) -> ("Config"=w58:string[][])
        n9 = call "Index_Config.vi"("Action"="BOOST_MODE_Orifice_size", "config"=w58) -> ("data"=w54:string)  [unwired: 9 in]
        n10 = disable-structure shown="禁用" {
          disable-tunnel: w61 -> [w76 _]
          disable-tunnel: [w75 _] -> w60
          disable-tunnel: [w69 _] -> w59
          disable-tunnel: w54 -> [w68 _]
          frame Disabled {
            n11 = Unbundle By Name(w76) -> ("Motor.COM"=w81:refnum<visa-resource-name>)
            n12 = call "Position_Config.vi"("Step"=enum16{"Initial", "Write", "Read"}."Read") -> ("Position Config out"=w78:T8)  [unwired: 9 in, 1 out]
            n13 = case shown="\"12.7\", Default" w68 {
              tunnel: w78 -> [w88 w90 w92 w94]
              tunnel: [w87 w89 w91 w93] -> w77
              frame "12.7", Default {
                n14 = Unbundle By Name(w88) -> ("OrificeSize_12.7"=w87:i32)
              }
              frame "13" {
                n15 = Unbundle By Name(w90) -> ("OrificeSize_13"=w89:i32)
              }
              frame "30" {
                n16 = Unbundle By Name(w92) -> ("OrificeSize_30"=w91:i32)
              }
              frame "16" {
                n17 = Unbundle By Name(w94) -> ("OrificeSize_16"=w93:i32)
              }
            }
            n18 = call "IO.vi"("DO DATA"=bool[] [FALSE] ("Writel_IO"), "IO Name"=string[] ["Orifice_fixed_Cylinder"], "IO?"=enum16{"DI", "DO"}."DO") -> ("error out"=w71:errorcluster)  [unwired: 7 in, 1 out]
            n19 = To Long Integer(number=w77) -> (32bit integer=w83:i32)
            n20 = call "Time Delay"("error in (no error)"=w71) -> ("error out"=w70:errorcluster)  [unwired: 10 in]
            n21 = call "Pulse.vi"("Pulse"=w83) -> ("Pulse"=w84:string)  [unwired: 10 in]
            n22 = call "Motor Visa.vi"("错误输入（无错误）"=w70, "Command"=w84, "VISA资源名称"=w81) -> ("错误输出"=w85:errorcluster, "VISA资源名称输出"=w86:refnum<visa-resource-name>)  [unwired: 6 in, 1 out]
            n23 = call "ABS.vi"() -> ("绝对模式"=w82:string)  [unwired: 11 in]
            n24 = call "Motor Visa.vi"("错误输入（无错误）"=w85, "Command"=w82, "VISA资源名称"=w86) -> ("VISA资源名称输出"=w80:refnum<visa-resource-name>)  [unwired: 6 in, 2 out]
            n25 = while {
              tunnel: w80 -> [w120]
              tunnel: [w103] -> w75
              stop <- w110 stop-if-true
              n26 = call "Get Status.vi"() -> ("Command"=w121:string)  [unwired: 11 in]
              n27 = call "Get Alarm  Error Status.vi"() -> ("AlarmStatus"=w113:string, "ErrorStatus"=w114:string)  [unwired: 10 in]
              n28 = call "Motor Visa.vi"("Command"=w121, "VISA资源名称"=w120) -> ("读取缓冲区"=w119:string, "VISA资源名称输出"=w112:refnum<visa-resource-name>)  [unwired: 7 in, 1 out]
              n29 = Wait (ms)(milliseconds to wait=u32 50 ("等待时间（毫秒）")) -> ()  [unwired: 1 out]
              n30 = call "Motor Visa.vi"("Command"=w114, "VISA资源名称"=w112) -> ("读取缓冲区"=w116:string, "VISA资源名称输出"=w117:refnum<visa-resource-name>)  [unwired: 7 in, 1 out]
              n31 = call "Motor Visa.vi"("Command"=w113, "VISA资源名称"=w117) -> ("读取缓冲区"=w115:string)  [unwired: 7 in, 2 out]
              n32 = call "Exit.vi"("Step"=enum16{"Initial", "Write", "Read"}."Read" ("step")) -> ("Exit Out"=w106:bool)  [unwired: 9 in, 1 out]
              n33 = call "Stop.vi"("Step"=enum16{"Initial", "Write", "Read"}."Read") -> ("Stop Out"=w107:bool)  [unwired: 9 in, 1 out]
              n34 = call "Alarm and Error Result.vi"("Command"=w115) -> ("Alarm or Error"=w105:bool)  [unwired: 10 in]
              n35 = call "Alarm and Error Result.vi"("Command"=w116) -> ("Alarm or Error"=w104:bool)  [unwired: 10 in]
              n36 = call "Motion Down.vi"("Command"=w119) -> ("Motion Down"=w111:bool)  [unwired: 10 in]
              n37 = Compound Arithmetic op=OR(w106, w107, w105, w104, w111) -> (w110:bool)
              n38 = Or(x=w105, y=w104) -> (x .or. y?=w103:bool)
            }
            n39 = case shown="True" w75 {
              tunnel: [_ "Error" ("Message Name")] -> w69
              frame False {
                n40 = call "IO.vi"("DO DATA"=bool[] [TRUE] ("Writel_IO"), "IO Name"=string[] ["Orifice_fixed_Cylinder"], "IO?"=enum16{"DI", "DO"}."DO") -> ("error out"=w98:errorcluster)  [unwired: 7 in, 1 out]
                n41 = call "Time Delay2"("error in (no error)"=w98) -> ()  [unwired: 10 in, 1 out]
              }
              frame True {
                n42 = call "6-AlarmStatus.vi"("AlarmValue"=TRUE, "AlarmIndex"=AlarmIndex."Motor Error", "Step"=enum16{"Initial", "Write", "Read"}."Write") -> ()  [unwired: 7 in, 2 out]
              }
            }
          }
          frame Enabled {
          }
        }
        n43 = call "LogStatus.vi"("error in (no error)"=w66, "last message"=w64, "message"=w63) -> ("error  out"=w65:errorcluster)  [unwired: 8 in]
        n44 = Bundle By Name(cluster=w53, "BOOST.Restriction Plate Diameter"=w54, "BOOST_Status.Restriction Plate Diameter"="PASS") -> (w55:T2)
      }
      frame "BOOST_Motor_On_with_power_mode" {
        n45 = Unbundle By Name(w125) -> ("Table"=w133:string[][], "daemon reference"=w138:refnum<k5>, "Config"=w131:string[][])
        n46 = call "Select_Table_Vaule Enable_Disable.vi"("Action"=w134, "Table"=w133) -> ("Enable"=w135:bool)  [unwired: 8 in, 1 out]
        n47 = case shown="True" w135 {
          tunnel: w138 -> [w145 w163]
          tunnel: [TRUE w153] -> _
          tunnel: [w145 w157] -> w122
          tunnel: ["" ("response") w149] -> w127
          tunnel: w134 -> [_ w156]
          tunnel: w133 -> [_ w155]
          tunnel: w131 -> [_ w152]
          tunnel: "BOOST_MODE_Drive_mode" -> [_ w151]
          tunnel: [_ w150] -> w124
          tunnel: [_ w149] -> _
          tunnel: [_ w148] -> _
          tunnel: [_ w147] -> _
          frame False {
          }
          frame True {
            (unwired) "B2" ("Power Mode")
            w162 = "UIdisplay" ("Process (\"\" - local)")
            n48 = call "Index_Config.vi"("Action"=w151, "config"=w152) -> ("data"=w147:string)  [unwired: 9 in]
            n49 = call "drive_motor.vi"("Power Mode"=w147, "daemon reference in"=w163) -> ("error out"=w150:errorcluster, "response"=w149:string, "daemon reference out"=w157:refnum<k5>)  [unwired: 6 in, 1 out]
            n50 = call "Select_Table_Vaule.vi"("Vaule"=w149, "Action"=w156, "Table"=w155) -> ("Result"=w153:bool, "vaule"=w154:string[])  [unwired: 7 in]
            n51 = Append True/False String(1:w153, 2:"FAIL" ("真字符串"), 3:"PASS" ("真字符串")) -> (0:w148:string)  [unwired: 1 in]
            n52 = Build Array (concatenate)(w154, w149, w148) -> (w161:string[])
            n53 = Flatten To XML(anything=w161) -> (xml string=w160:string)
            n54 = call "AMC Send Local Message.vi"("Process (\"\" - local)"=w162, "Message Value"=w160, "Message Name"=w162) -> ()  [unwired: 7 in, 2 out]
          }
        }
        n55 = call <vilib>:"Space Constant.vi"() -> ("String"=w137:string)
        n56 = Concatenate Strings(w134, w137, w127) -> (w136:string)
        n57 = Bundle By Name(cluster=w125, "daemon reference"=w122) -> (w123:T2)
        n58 = call "LogStatus.vi"("error in (no error)"=w124, "last message"=w139, "message"=w136) -> ("error  out"=w140:errorcluster)  [unwired: 8 in]
        n59 = case shown="Error" w124 {
          tunnel: [_ TRUE] -> w128
          tunnel: [_ "Error"] -> w129
          frame No Error {
          }
          frame Error {
          }
        }
      }
      frame "BOOST_Wait_for_X_sec_for_motor_speed_to_stabilise" {
        # "来之Config"
        n60 = Unbundle By Name(w169) -> ("Config"=w172:string[][])
        n61 = Get Date/Time In Seconds() -> (seconds since 1Jan1904=w166:timestamp)
        n62 = call "Index_Config.vi"("Action"="BOOST_MODE_Stabilisation_time", "config"=w172) -> ("data"=w167:string)  [unwired: 9 in]
        n63 = Fract/Exp String To Number(string=w167) -> (number=w165:dbl)  [unwired: 3 in, 1 out]
        n64 = while {
          tunnel: w166 -> [w187]
          tunnel: w165 -> [w184]
          tunnel: [w183] -> _
          stop <- w183 stop-if-true
          n65 = Get Date/Time In Seconds() -> (seconds since 1Jan1904=w188:timestamp)
          n66 = Subtract(x=w188, y=w187) -> (x-y=w186:dbl)
          n67 = call "6-AlarmStatus.vi"("Step"=enum16{"Initial", "Write", "Read"}."Read") -> ("AlarmValue Out"=w191:bool[])  [unwired: 9 in, 1 out]
          n68 = Greater Or Equal?(x=w186, y=w184) -> (x >= y?=w185:bool)
          n69 = call "Stop.vi"("Step"=enum16{"Initial", "Write", "Read"}."Read") -> ("Stop Out"=w189:bool)  [unwired: 9 in, 1 out]
          n70 = call "Exit.vi"("Step"=enum16{"Initial", "Write", "Read"}."Read" ("step")) -> ("Exit Out"=w193:bool)  [unwired: 9 in, 1 out]
          n71 = Or Array Elements(Boolean array=w191) -> (logical OR=w190:bool)
          n72 = Compound Arithmetic op=OR(w185, w189, w193, w190) -> (w183:bool)
          n73 = Wait (ms)(milliseconds to wait=u32 1 ("等待时间（毫秒）")) -> ()  [unwired: 1 out]
        }
        n74 = Search and Replace String(input string=w174, search string="X" ("搜索字符串"), replace string=w167) -> (result string=w175:string)  [unwired: 5 in, 3 out]
        n75 = call "LogStatus.vi"("error in (no error)"=w179, "last message"=w177, "message"=w175) -> ("error  out"=w178:errorcluster)  [unwired: 8 in]
        n76 = Bundle By Name(cluster=w169, "BOOST.BOOST - Stabilisation Time"=w167, "BOOST_Status.BOOST - Stabilisation Time"="PASS") -> (w168:T2)
      }
      frame "BOOST_Get_and_check_DDM_Parameter" {
        n77 = Unbundle By Name(w211) -> ("Table"=w224:string[][], "daemon reference"=w231:refnum<k5>, "Config"=w222:string[][])
        n78 = call "Select_Table_Vaule Enable_Disable.vi"("Action"=w225, "Table"=w224) -> ("Enable"=w223:bool)  [unwired: 8 in, 1 out]
        n79 = case shown="False" w223 {
          tunnel: w231 -> [w240 w266]
          tunnel: [w240 w265] -> w210
          tunnel: [w239 w257] -> w226
          tunnel: w225 -> [_ w262]
          tunnel: w224 -> [_ w267]
          tunnel: w222 -> [_ _]
          tunnel: [_ w251] -> w220
          tunnel: [_ w264] -> w219
          tunnel: [_ w255] -> w212
          tunnel: T7[] ["voltage", "current", "power", "speed", "measured_power", "pressure", "lsi_magnet_temp", "fisf_magnet_temp", "iir_magnet_temp"] ("Parameter") -> [_ w250]
          tunnel: [w238 w242] -> w208
          tunnel: [w238 w241] -> w201
          frame False {
            w239 = "Skip" ("software string")
            n80 = Initialize Array(w239, 6 ("维数大小")) -> (w238:string[])
          }
          frame True {
            w256 = string[] ["BOOST_DDM_Voltage", "BOOST_DDM_Current", "BOOST_DDM_Power", "BOOST_DDM_Speed", "BOOST_DDM_Measured_Power", "BOOST_DDM_Pressure", "BOOST_lsi_magnet_temp", "BOOST_fisf_magnet_temp", "BOOST_iir_magnet_temp"]
            n81 = for {
              tunnel: [w273] -> w249 mode=indexing
              tunnel: [w272] -> w255
              tunnel: [w268] -> w252 mode=indexing
              tunnel: w250 -> [w270] mode=indexing
              shift-right: [w274] -> w265
              shift-left: w266 -> [w275]
              n82 = Build Array(w270) -> (w269:T7[])
              n83 = call "get_parameter.vi"("Parameter"=w269, "daemon reference in"=w275) -> ("error out"=w272:errorcluster, "response"=w273:string, "values"=w271:dbl[], "daemon reference out"=w274:refnum<k5>)  [unwired: 5 in, 1 out]
              n84 = Index Array(array=w271) -> (element=w268:dbl)  [unwired: 1 in]
            }
            n85 = in-place {
              w280 = 1000.0
              n86 = in-place-array #1(w252, 3, 5) -> (w279:dbl, w276:dbl)
              n87 = Divide(x=w279, y=w280) -> (x/y=w278:dbl)
              n88 = Divide(x=w276, y=w280) -> (x/y=w277:dbl)
              n89 = in-place-array #1(w278, w277) -> (w251:dbl[])  [unwired: 2 out]
            }
            n90 = Array To Spreadsheet String(delimiter (Tab)=",", array=w249, 3:"" ("format string")) -> (spreadsheet string=w248:string)
            n91 = Number To Fractional String(number=w251) -> (F-format string=w242:string[])  [unwired: 3 in]
            n92 = Interleave 1D Arrays(w256, w242) -> (w258:string[])
            n93 = Array To Spreadsheet String(delimiter (Tab)=";" ("分隔符(Tab)"), array=w258, 3:"" ("格式字符串")) -> (spreadsheet string=w257:string)
            n94 = Build Array (concatenate)(w262, w256) -> (w263:string[])
            n95 = Build Array (concatenate)(w248, w242) -> (w261:string[])
            n96 = for {
              tunnel: w267 -> [w287]
              tunnel: w261 -> [w285] mode=indexing
              tunnel: w263 -> [w284] mode=indexing
              tunnel: [w283] -> w264 mode=indexing
              tunnel: [w281] -> w243 mode=indexing
              w292 = "UIdisplay" ("Process (\"\" - local)")
              n97 = call "Select_Table_Vaule.vi"("Boolean"=TRUE, "Vaule"=w285, "Action"=w284, "Table"=w287) -> ("Result"=w283:bool, "vaule"=w286:string[])  [unwired: 6 in]
              n98 = Append True/False String(1:w283, 2:"FAIL" ("真字符串"), 3:"PASS" ("真字符串")) -> (0:w281:string)  [unwired: 1 in]
              n99 = Build Array (concatenate)(w286, w285, w281) -> (w291:string[])
              n100 = Flatten To XML(anything=w291) -> (xml string=w290:string)
              n101 = call "AMC Send Local Message.vi"("Process (\"\" - local)"=w292, "Message Value"=w290, "Message Name"=w292) -> ()  [unwired: 7 in, 2 out]
            }
            n102 = Delete From Array(array=w243, length=1 ("长度"), index=0 ("索引")) -> (array with subset deleted=w241:string[])  [unwired: 1 out]
          }
        }
        n103 = call <vilib>:"Space Constant.vi"() -> ("String"=w228:string)
        n104 = Concatenate Strings(w225, w228, w226) -> (w227:string)
        n105 = Index Array(array=w201) -> (element #1=w200:string, element #2=w199:string, element #3=w198:string, element #4=w196:string, element #5=w197:string, element #6=w195:string)  [unwired: 6 in]
        n106 = Index Array(array=w208) -> (element #1=w207:string, element #2=w206:string, element #3=w205:string, element #4=w204:string, element #5=w203:string, element #6=w202:string)  [unwired: 6 in]
        n107 = Bundle By Name(cluster=w211, "daemon reference"=w210, "BOOST.BOOST - DDM Parameter - Voltage"=w207, "BOOST.BOOST - DDM Parameter - Current"=w206, "BOOST.BOOST - DDM Parameter - Power"=w205, "BOOST.BOOST - DDM Parameter - Measured Power"=w203, "BOOST.BOOST - DDM Parameter - Speed"=w204, "BOOST.BOOST - DDM Parameter - Pressure"=w202, "BOOST_Status.BOOST - DDM Parameter - Voltage"=w200, "BOOST_Status.BOOST - DDM Parameter - Current"=w199, "BOOST_Status.BOOST - DDM Parameter - Power"=w198, "BOOST_Status.BOOST - DDM Parameter - Measured Power"=w197, "BOOST_Status.BOOST - DDM Parameter - Speed"=w196, "BOOST_Status.BOOST - DDM Parameter - Pressure"=w195) -> (w209:T2)
        n108 = call "LogStatus.vi"("error in (no error)"=w212, "last message"=w232, "message"=w227) -> ("error  out"=w233:errorcluster)  [unwired: 8 in]
        n109 = Delete From Array(array=w219, length=1 ("长度"), index=0 ("索引")) -> (array with subset deleted=w218:bool[])  [unwired: 1 out]
        n110 = Bundle By Name(cluster=w230, "BOOST.DDM_Parameter"=w220, "BOOST.DDM_Parameter_status"=w218) -> (w229:T3)
        n111 = case shown="Error" w212 {
          tunnel: [_ TRUE] -> w214
          tunnel: [_ "Error"] -> w215
          frame No Error {
          }
          frame Error {
          }
        }
      }
      frame "BOOST_Get_and_check_tester_Parameter" {
        w309 = "BOOST_Calculate_and_check_tester_parameter"
        n112 = Unbundle By Name(w325) -> ("Table"=w338:string[][], "daemon reference"=w344:refnum<k5>, "Config"=w336:string[][])
        n113 = call "Select_Table_Vaule Enable_Disable.vi"("Action"=w339, "Table"=w338) -> ("Enable"=w337:bool)  [unwired: 8 in, 1 out]
        n114 = case shown="False" w337 {
          tunnel: w344 -> [w352 w369]
          tunnel: [w352 w369] -> w324
          tunnel: [w351 w360] -> w340
          tunnel: w339 -> [_ w366]
          tunnel: w338 -> [_ w370]
          tunnel: w336 -> [_ _]
          tunnel: [_ w358] -> w330
          tunnel: [_ w368] -> w329
          tunnel: [w350 w354] -> w323
          tunnel: [w350 w353] -> w299
          frame False {
            w351 = "Skip" ("software string")
            n115 = Initialize Array(w351, 6 ("维数大小")) -> (w350:string[])
          }
          frame True {
            w359 = string[] ["BOOST_PM_Voltage", "BOOST_PM_Current", "BOOST_PM_Power", "BOOST_Ambient_Pressure", "BOOST_Ambient_Temperature", "BOOST_Ambient_humidity", "BOOST_Tester_Reference_Ambient_Pressure"]
            n116 = call "Power_Tunings_Tester_Parameter.vi"() -> ("Power_Tuning_Tester_Parameter"=w358:dbl[])  [unwired: 11 in]
            n117 = Number To Fractional String(number=w358) -> (F-format string=w354:string[])  [unwired: 3 in]
            n118 = Interleave 1D Arrays(w359, w354) -> (w361:string[])
            n119 = Array To Spreadsheet String(delimiter (Tab)=";" ("分隔符(Tab)"), array=w361, 3:"" ("格式字符串")) -> (spreadsheet string=w360:string)
            n120 = Build Array (concatenate)(w366, w359) -> (w367:string[])
            n121 = Build Array (concatenate)("", w354) -> (w365:string[])
            n122 = for {
              tunnel: w370 -> [w377]
              tunnel: w365 -> [w375] mode=indexing
              tunnel: w367 -> [w374] mode=indexing
              tunnel: [w373] -> w368 mode=indexing
              tunnel: [w371] -> w355 mode=indexing
              w382 = "UIdisplay" ("Process (\"\" - local)")
              n123 = call "Select_Table_Vaule.vi"("Boolean"=TRUE, "Vaule"=w375, "Action"=w374, "Table"=w377) -> ("Result"=w373:bool, "vaule"=w376:string[])  [unwired: 6 in]
              n124 = Append True/False String(1:w373, 2:"FAIL" ("真字符串"), 3:"PASS" ("真字符串")) -> (0:w371:string)  [unwired: 1 in]
              n125 = Build Array (concatenate)(w376, w375, w371) -> (w381:string[])
              n126 = Flatten To XML(anything=w381) -> (xml string=w380:string)
              n127 = call "AMC Send Local Message.vi"("Process (\"\" - local)"=w382, "Message Value"=w380, "Message Name"=w382) -> ()  [unwired: 7 in, 2 out]
            }
            n128 = Delete From Array(array=w355, length=1 ("长度"), index=0 ("索引")) -> (array with subset deleted=w353:string[])  [unwired: 1 out]
          }
        }
        n129 = call <vilib>:"Space Constant.vi"() -> ("String"=w342:string)
        n130 = Unbundle By Name(w313) -> ("MES bool"=w318:refnum<vi>)
        n131 = call "HD_Config.vi"("Step"=enum16{"Initial", "Write", "Read"}."Read") -> ("HD Config out"=w319:T5)  [unwired: 9 in, 1 out]
        n132 = property class="Bool (严格)"(reference=w318) -> ("Value"=w316:bool)  [unwired: 1 in, 2 out]
        n133 = Unbundle By Name(w319) -> ("GRR"=w308:bool, "Fail_resume_mode"=w317:bool)
        n134 = Concatenate Strings(w339, w342, w340) -> (w341:string)
        n135 = Not(x=w316) -> (.not. x?=w314:bool)
        n136 = Or(x=w317, y=w314) -> (x .or. y?=w315:bool)
        n137 = Index Array(array=w299) -> (element #1=w298:string, element #2=w297:string, element #3=w296:string, element #4=w295:string, element #5=w294:string, element #6=w293:string)  [unwired: 6 in]
        n138 = Index Array(array=w323) -> (element #1=w305:string, element #2=w304:string, element #3=w303:string, element #4=w302:string, element #5=w301:string, element #6=w300:string)  [unwired: 6 in]
        n139 = Unbundle By Name(w334) -> ("BOOST.DDM_Parameter_status"=w333:bool[])
        n140 = Bundle By Name(cluster=w325, "daemon reference"=w324, "BOOST.BOOST - Tester Parameter - Voltage"=w305, "BOOST.BOOST - Tester Parameter - Current"=w304, "BOOST.BOOST - Tester Parameter - Power"=w303, "BOOST.BOOST - Tester Parameter - Ambient Pressure"=w302, "BOOST.BOOST - Tester Parameter - Ambient Temperature"=w301, "BOOST.BOOST - Tester Parameter - Ambient Humidity"=w300, "BOOST_Status.BOOST - Tester Parameter - Voltage"=w298, "BOOST_Status.BOOST - Tester Parameter - Current"=w297, "BOOST_Status.BOOST - Tester Parameter - Power"=w296, "BOOST_Status.BOOST - Tester Parameter - Ambient Pressure"=w295, "BOOST_Status.BOOST - Tester Parameter - Ambient Temperature"=w294, "BOOST_Status.BOOST - Tester Parameter - Ambient Humidity"=w293) -> (w322:T2)
        n141 = Delete From Array(array=w329, length=1 ("长度"), index=0 ("索引")) -> (array with subset deleted=w328:bool[])  [unwired: 1 out]
        n142 = Build Array (concatenate)(w333, w328) -> (w332:bool[])
        n143 = And Array Elements(Boolean array=w332) -> (logical AND=w312:bool)
        n144 = call "LogStatus.vi"("error in (no error)"=w347, "last message"=w345, "message"=w341) -> ("error  out"=w346:errorcluster)  [unwired: 8 in]
        n145 = Select(t=TRUE, s=w315, f=w312) -> (s? t:f=w307:bool)
        n146 = Bundle By Name(cluster=w334, "BOOST.Get_Tester_Parameter"=w330, "BOOST.Get_Tester_Parameter_status"=w328) -> (w343:T3)
        n147 = Select(t=w309, s=w307, f="Finalization_NG_unit") -> (s? t:f=w311:string)
        n148 = Select(t=w308, s=w308, f=w307) -> (s? t:f=w306:bool)
        n149 = Select(t=w309, s=w308, f=w311) -> (s? t:f=w310:string)
        n150 = Not(x=w306) -> (.not. x?=w331:bool)
      }
      frame "BOOST_Calculate_and_check_tester_parameter" {
        n151 = Unbundle By Name(w417) -> ("BOOST.DDM_Parameter"=w412:dbl[], "BOOST.Get_Tester_Parameter"=w411:dbl[])
        n152 = Unbundle By Name(w403) -> ("Table"=w406:string[][], "daemon reference"=w405:refnum<k5>, "Config"=w404:string[][])
        n153 = Unbundle By Name(w407) -> ("FCO.COM"=w409:refnum<visa-resource-name>)
        n154 = call "Index_Config.vi"("Action"="BOOST_MODE_Orifice_size", "config"=w404) -> ("data"=w410:string)  [unwired: 9 in]
        n155 = call "Select_Table_Vaule Enable_Disable.vi"("Action"=w420, "Table"=w406) -> ("Enable"=w419:bool)  [unwired: 8 in, 1 out]
        n156 = case shown="False" w419 {
          tunnel: w405 -> [w432 w457]
          tunnel: [w432 w457] -> w400
          tunnel: [w431 w448] -> w421
          tunnel: w420 -> [_ w454]
          tunnel: w406 -> [_ w458]
          tunnel: [_ w440] -> w418
          tunnel: [_ w456] -> w416
          tunnel: w412 -> [_ w444]
          tunnel: w411 -> [_ w443]
          tunnel: w410 -> [_ w442]
          tunnel: w409 -> [_ w441]
          tunnel: [w430 w436] -> w401
          tunnel: [w430 w435] -> w388
          tunnel: [_ w433] -> _
          frame False {
            w431 = "Skip" ("software string")
            n157 = Initialize Array(w431, 5 ("维数大小")) -> (w430:string[])
          }
          frame True {
            w447 = string[] ["BOOST_DDM_Pressure_corrected", "BOOST_DDM_Real_Power", "BOOST_Delta_V", "BOOST_Flow_rate", "BOOST_AW"]
            n158 = call "FCO_Read.vi"("VISA in"=w441) -> ("Pressure(Pa)"=w434:dbl)  [unwired: 7 in, 3 out]
            n159 = Fract/Exp String To Number(string=w442) -> (number=w446:dbl)  [unwired: 3 in, 1 out]
            n160 = call "AW_Calculate_Tester_Parameter.vi"("Tester Parameter"=w443, "DDM Parameter"=w444, "AW_Box_Pressure/Stag Total-Static Pressure rise"=w434, "Orifice_Plate_Diameter"=w446) -> ("Calculate Tester Parameter"=w445:dbl[])  [unwired: 7 in]
            n161 = Number To Fractional String(number=w445) -> (F-format string=w436:string[])  [unwired: 3 in]
            n162 = Number To Fractional String(number=w434) -> (F-format string=w433:string)  [unwired: 3 in]
            n163 = Interleave 1D Arrays(w447, w436) -> (w451:string[])
            n164 = Array To Spreadsheet String(delimiter (Tab)=";" ("分隔符(Tab)"), array=w451, 3:"" ("格式字符串")) -> (spreadsheet string=w448:string)
            n165 = Build Array (concatenate)(w454, w447) -> (w455:string[])
            n166 = Build Array (concatenate)("", w436) -> (w453:string[])
            n167 = for {
              tunnel: w458 -> [w464]
              tunnel: w453 -> [w462] mode=indexing
              tunnel: w455 -> [w461] mode=indexing
              tunnel: [w460] -> w456 mode=indexing
              tunnel: [w459] -> w437 mode=indexing
              w469 = "UIdisplay" ("Process (\"\" - local)")
              n168 = call "Select_Table_Vaule.vi"("Vaule"=w462, "Action"=w461, "Table"=w464) -> ("Result"=w460:bool, "vaule"=w463:string[])  [unwired: 7 in]
              n169 = Append True/False String(1:w460, 2:"FAIL" ("真字符串"), 3:"PASS" ("真字符串")) -> (0:w459:string)  [unwired: 1 in]
              n170 = Build Array (concatenate)(w463, w462, w459) -> (w468:string[])
              n171 = Flatten To XML(anything=w468) -> (xml string=w467:string)
              n172 = call "AMC Send Local Message.vi"("Process (\"\" - local)"=w469, "Message Value"=w467, "Message Name"=w469) -> ()  [unwired: 7 in, 2 out]
            }
            n173 = Build Array (concatenate)(w445, w434) -> (w440:dbl[])
            n174 = Delete From Array(array=w437, length=1 ("长度"), index=0 ("索引")) -> (array with subset deleted=w435:string[])  [unwired: 1 out]
          }
        }
        n175 = call <vilib>:"Space Constant.vi"() -> ("String"=w423:string)
        n176 = Concatenate Strings(w420, w423, w421) -> (w422:string)
        n177 = Index Array(array=w388) -> (element #1=w387:string, element #2=w386:string, element #3=w385:string, element #4=w384:string, element #5=w383:string)  [unwired: 5 in]
        n178 = Index Array(array=w401) -> (element #1=w393:string, element #2=w392:string, element #3=w391:string, element #4=w390:string, element #5=w389:string)  [unwired: 5 in]
        n179 = Bundle By Name(cluster=w403, "daemon reference"=w400, "BOOST.BOOST - Calculated Parameter - DDM Pressure Corrected"=w393, "BOOST.BOOST - Calculated Parameter - DDM Real Power"=w392, "BOOST.BOOST - Calculated Parameter - Delta V"=w391, "BOOST.BOOST - Calculated Parameter - Flowrate"=w390, "BOOST.BOOST - Calculated Parameter - Airwatt"=w389, "BOOST_Status.BOOST - Calculated Parameter - DDM Pressure Corrected"=w387, "BOOST_Status.BOOST - Calculated Parameter - DDM Real Power"=w386, "BOOST_Status.BOOST - Calculated Parameter - Delta V"=w385, "BOOST_Status.BOOST - Calculated Parameter - Flowrate"=w384, "BOOST_Status.BOOST - Calculated Parameter - Airwatt"=w383) -> (w402:T2)
        n180 = call "HD_Config.vi"("Step"=enum16{"Initial", "Write", "Read"}."Read") -> ("HD Config out"=w398:T5)  [unwired: 9 in, 1 out]
        n181 = Unbundle By Name(w398) -> ("GRR"=w394:bool)
        n182 = call "LogStatus.vi"("error in (no error)"=w427, "last message"=w425, "message"=w422) -> ("error  out"=w426:errorcluster)  [unwired: 8 in]
        n183 = Delete From Array(array=w416, length=1 ("长度"), index=0 ("索引")) -> (array with subset deleted=w415:bool[])  [unwired: 1 out]
        n184 = Bundle By Name(cluster=w417, "BOOST.Cal_Tester_Parameter"=w418, "BOOST.Cal_Tester_Parameter_status"=w415) -> (w424:T3)
        n185 = Select(t="Airwatts_Tunings_&_Performance_Test_Max_Power_MODE", s=w394, f="BOOST_Air_Muscle_Check") -> (s? t:f=w395:string)
      }
      frame "BOOST_Air_Muscle_Check" {
        w494 = "UIdisplay" ("Process (\"\" - local)")
        n186 = Unbundle By Name(w470) -> ("MES bool"=w477:refnum<vi>)
        n187 = call "HD_Config.vi"("Step"=enum16{"Initial", "Write", "Read"}."Read") -> ("HD Config out"=w478:T5)  [unwired: 9 in, 1 out]
        n188 = Unbundle By Name(w497) -> ("BOOST.Cal_Tester_Parameter_status"=w495:bool[])
        n189 = property class="Bool (严格)"(reference=w477) -> ("Value"=w475:bool)  [unwired: 1 in, 2 out]
        n190 = Unbundle By Name(w478) -> ("Fail_resume_mode"=w476:bool)
        n191 = Unbundle By Name(w472) -> ("Table"=w480:string[][])
        n192 = Not(x=w475) -> (.not. x?=w474:bool)
        n193 = Or(x=w476, y=w474) -> (x .or. y?=w473:bool)
        n194 = call "LogStatus.vi"("error in (no error)"=w505, "last message"=w504, "message"=w486) -> ("error  out"=w503:errorcluster)  [unwired: 8 in]
        n195 = call "Select_Table_Vaule Enable_Disable.vi"("Action"=w486, "Table"=w480) -> ("Enable"=w483:bool)  [unwired: 8 in, 1 out]
        n196 = case shown="True" w483 {
          tunnel: w503 -> [w524 w543]
          tunnel: [w524 w542] -> w502
          tunnel: w501 -> [w526 w541]
          tunnel: [w526 w540] -> w500
          tunnel: [w525 w539] -> w499
          tunnel: [w514 w531] -> w498
          tunnel: w497 -> [w525 w538]
          tunnel: [w513 w534] -> w496
          tunnel: w495 -> [w517 _]
          tunnel: w473 -> [w509 _]
          tunnel: w472 -> [w506 w529]
          tunnel: [w506 w528] -> w471
          tunnel: w470 -> [_ w527]
          frame False {
            n197 = And Array Elements(Boolean array=w517) -> (logical AND=w508:bool)
            n198 = Index Array(array=w517, index=1 ("索引")) -> (element=w518:bool)
            n199 = Select(t=TRUE, s=w509, f=w508) -> (s? t:f=w507:bool)
            n200 = Select(t="BOOST_Stop_motor", s=w507, f="Finalization_NG_unit") -> (s? t:f=w520:string)
            n201 = Select(t=w520, s=w518, f="BOOST_Power_Tune") -> (s? t:f=w514:string)
            n202 = Equal?(x=w514, y="Finalization_NG_unit") -> (x = y?=w512:bool)
            n203 = Equal?(x=w514, y="Error") -> (x = y?=w511:bool)
            n204 = Or(x=w512, y=w511) -> (x .or. y?=w513:bool)
          }
          frame True {
            n205 = call "3.2.1_BOOST_Air_Muscle_Check.vi"("Data in"=w529, "error in (no error)"=w543, "AllControls In"=w527, 10:w538, "Message Queue out"=w541) -> ("error out"=w542:errorcluster, "Flow"=w531:string, "Data"=w539:T3, "Message Queue Out"=w540:T4, "Data out"=w528:T2)  [unwired: 2 in]
            n206 = Equal?(x=w531, y="Finalization_NG_unit") -> (x = y?=w536:bool)
            n207 = Equal?(x=w531, y="Error") -> (x = y?=w533:bool)
            n208 = Equal?(x=w531, y="BOOST_Stop_motor") -> (x = y?=w530:bool)
            n209 = Compound Arithmetic op=OR(w536, w533, w530) -> (w534:bool)
          }
        }
        n210 = Select(t="Enable" ("元素"), s=w483, f="Disable" ("元素")) -> (s? t:f=w482:string)
        n211 = call "Select_Table_Vaule.vi"("Vaule"=w482, "Action"=w486, "Table"=w480) -> ("Result"=w487:bool, "vaule"=w488:string[])  [unwired: 7 in]
        n212 = Append True/False String(1:w487, 2:"FAIL" ("真字符串"), 3:"PASS" ("真字符串")) -> (0:w489:string)  [unwired: 1 in]
        n213 = Build Array (concatenate)(w488, w482, w489) -> (w491:string[])
        n214 = Flatten To XML(anything=w491) -> (xml string=w490:string)
        n215 = call "AMC Send Local Message.vi"("Process (\"\" - local)"=w494, "Message Value"=w490, "Message Name"=w494) -> ()  [unwired: 7 in, 2 out]
        n216 = Flush Queue(queue=w500) -> (queue out=w481:T4)  [unwired: 1 in, 2 out]
      }
      frame "BOOST_Power_Tune" {
        w569 = "UIdisplay" ("Process (\"\" - local)")
        n217 = Unbundle By Name(w544) -> ("MES bool"=w551:refnum<vi>)
        n218 = call "HD_Config.vi"("Step"=enum16{"Initial", "Write", "Read"}."Read") -> ("HD Config out"=w552:T5)  [unwired: 9 in, 1 out]
        n219 = Unbundle By Name(w546) -> ("Table"=w561:string[][])
        n220 = property class="Bool (严格)"(reference=w551) -> ("Value"=w549:bool)  [unwired: 1 in, 2 out]
        n221 = Unbundle By Name(w552) -> ("Fail_resume_mode"=w550:bool)
        n222 = Not(x=w549) -> (.not. x?=w548:bool)
        n223 = call "Select_Table_Vaule Enable_Disable.vi"("Action"=w560, "Table"=w561) -> ("Enable"=w556:bool)  [unwired: 8 in, 1 out]
        n224 = Or(x=w550, y=w548) -> (x .or. y?=w547:bool)
        n225 = call "LogStatus.vi"("error in (no error)"=w578, "last message"=w577, "message"=w560) -> ("error  out"=w576:errorcluster)  [unwired: 8 in]
        n226 = case shown="True" w556 {
          tunnel: w576 -> [w584 w596]
          tunnel: [w584 w595] -> w575
          tunnel: w574 -> [w586 w594]
          tunnel: [w586 w593] -> w573
          tunnel: [w585 w592] -> w572
          tunnel: [w580 w590] -> w571
          tunnel: w570 -> [w585 w591]
          tunnel: w547 -> [w583 _]
          tunnel: w546 -> [w579 w589]
          tunnel: [w579 w588] -> w545
          tunnel: w544 -> [_ w587]
          frame False {
            n227 = Select(t="BOOST_Stop_motor", s=w583, f="Finalization_NG_unit") -> (s? t:f=w580:string)
          }
          frame True {
            n228 = call "3.2.2_BOOST_Power_Tune.vi"("Data in"=w589, "error in (no error)"=w596, "AllControls In"=w587, 10:w591, "Message Queue out"=w594) -> ("error out"=w595:errorcluster, "Flow"=w590:string, "Data"=w592:T3, "Message Queue Out"=w593:T4, "Data out"=w588:T2)  [unwired: 2 in]
          }
        }
        n229 = Select(t="Enable" ("元素"), s=w556, f="Disable" ("元素")) -> (s? t:f=w555:string)
        n230 = call "Select_Table_Vaule.vi"("Vaule"=w555, "Action"=w560, "Table"=w561) -> ("Result"=w562:bool, "vaule"=w563:string[])  [unwired: 7 in]
        n231 = Append True/False String(1:w562, 2:"FAIL" ("真字符串"), 3:"PASS" ("真字符串")) -> (0:w564:string)  [unwired: 1 in]
        n232 = Build Array (concatenate)(w563, w555, w564) -> (w566:string[])
        n233 = Flatten To XML(anything=w566) -> (xml string=w565:string)
        n234 = call "AMC Send Local Message.vi"("Process (\"\" - local)"=w569, "Message Value"=w565, "Message Name"=w569) -> ()  [unwired: 7 in, 2 out]
        n235 = Flush Queue(queue=w573) -> (queue out=w554:T4)  [unwired: 1 in, 2 out]
      }
    }
    n236 = call "6-AlarmStatus.vi"("Step"=enum16{"Initial", "Write", "Read"}."Read") -> ("AlarmValue Out"=w18:bool[])  [unwired: 9 in, 1 out]
    n237 = call "Stop.vi"("Step"=enum16{"Initial", "Write", "Read"}."Read") -> ("Stop Out"=w26:bool)  [unwired: 9 in, 1 out]
    n238 = call "Exit.vi"("Step"=enum16{"Initial", "Write", "Read"}."Read" ("step")) -> ("Exit Out"=w25:bool)  [unwired: 9 in, 1 out]
    n239 = Or Array Elements(Boolean array=w18) -> (logical OR=w17:bool)
    n240 = Compound Arithmetic op=OR(w24, w26, w25, w17) -> (w23:bool)
    n241 = call "AMC Run Step.vi"("Message Queue In"=w44, "Message Name"=w32, "Message Value"=w30, "error in (no error)"=w39, "Mli/Sig"=FALSE) -> ("Message Queue Out"=w43:T4, "error out"=w38:errorcluster)  [unwired: 13 in]
  }
  "Message Queue Out" <- w6
  "error out" <- w5
  "Data" <- w10
  "Flow" <- w7
  "Data out" <- w1
